vi "四台设备.vi"() -> ()   [LabVIEW 2012]
uses:
  <vilib>/Analysis/NI_AALPro.lvlib
panel:
  in  "选项卡控件 3":enum32{"振动", "振动 2", "转速", "温度湿度"}(tab)
  out "?":i16[](graph)
  out "?":i16[](graph)
  out "?":i16[](graph)
  out "?":i16[](graph)
  out "?":dbl[](graph)
  out "?":dbl[](graph)
  out "?":dbl[](graph)
  out "?":dbl[](graph)
  out "?":i16[](graph)
  out "?":dbl(graph)
  out "?":dbl(graph)
  out "?":dbl(graph)
  out "?":dbl(graph)
  out "?":u8(graph)
  out "?":u8(graph)
  out "?":dbl(graph)
  out "?":dbl(graph)
  in  "?":enum32{"振动", "振动 2", "转速", "温度湿度"}(tab)
  out "?":i16[](graph)
  out "?":i16[](graph)
  out "?":i16[](graph)
  out "?":i16[](graph)
  out "?":dbl[](graph)
  out "?":dbl[](graph)
  out "?":dbl[](graph)
  out "?":dbl[](graph)
  out "?":u16[](graph)
  out "?":dbl(graph)
  out "?":dbl(graph)
  out "?":u8(graph)
  out "?":dbl(graph)
  out "?":dbl(graph)
  out "?":u8(graph)
  out "?":dbl(graph)
  out "?":dbl(graph)
  in  "?":enum32{"振动", "振动 2", "转速", "温度湿度"}(tab)
  out "?":i16[](graph)
  out "?":i16[](graph)
  out "?":i16[](graph)
  out "?":i16[](graph)
  out "?":dbl[](graph)
  out "?":dbl[](graph)
  out "?":dbl[](graph)
  out "?":dbl[](graph)
  out "?":u16[](graph)
  out "?":dbl(graph)
  out "?":dbl(graph)
  out "?":dbl(graph)
  out "?":dbl(graph)
  out "?":dbl(graph)
  out "?":u8(graph)
  out "?":u8(graph)
  out "?":dbl(graph)
  out "KB/s 4":dbl
  out "收包 4":i32
  out "系统时间 4":string
  out "KB/s 3":dbl
  out "收包 3":i32
  out "系统时间 3":string
  out "KB/s 2":dbl
  out "收包 2":i32
  out "系统时间 2":string
  in  "?":enum32{"振动", "振动 2", "转速", "温度湿度"}(tab)
  out "?":i16[](graph)
  out "?":i16[](graph)
  out "?":i16[](graph)
  out "?":i16[](graph)
  out "?":dbl[](graph)
  out "?":dbl[](graph)
  out "?":dbl[](graph)
  out "?":dbl[](graph)
  out "?":u16[](graph)
  out "?":dbl(graph)
  out "?":dbl(graph)
  out "?":dbl(graph)
  out "?":dbl(graph)
  out "?":dbl(graph)
  out "?":dbl(graph)
  out "?":u8(graph)
  out "?":u8(graph)
  out "系统时间":string
  out "收包":i32
  out "KB/s":dbl
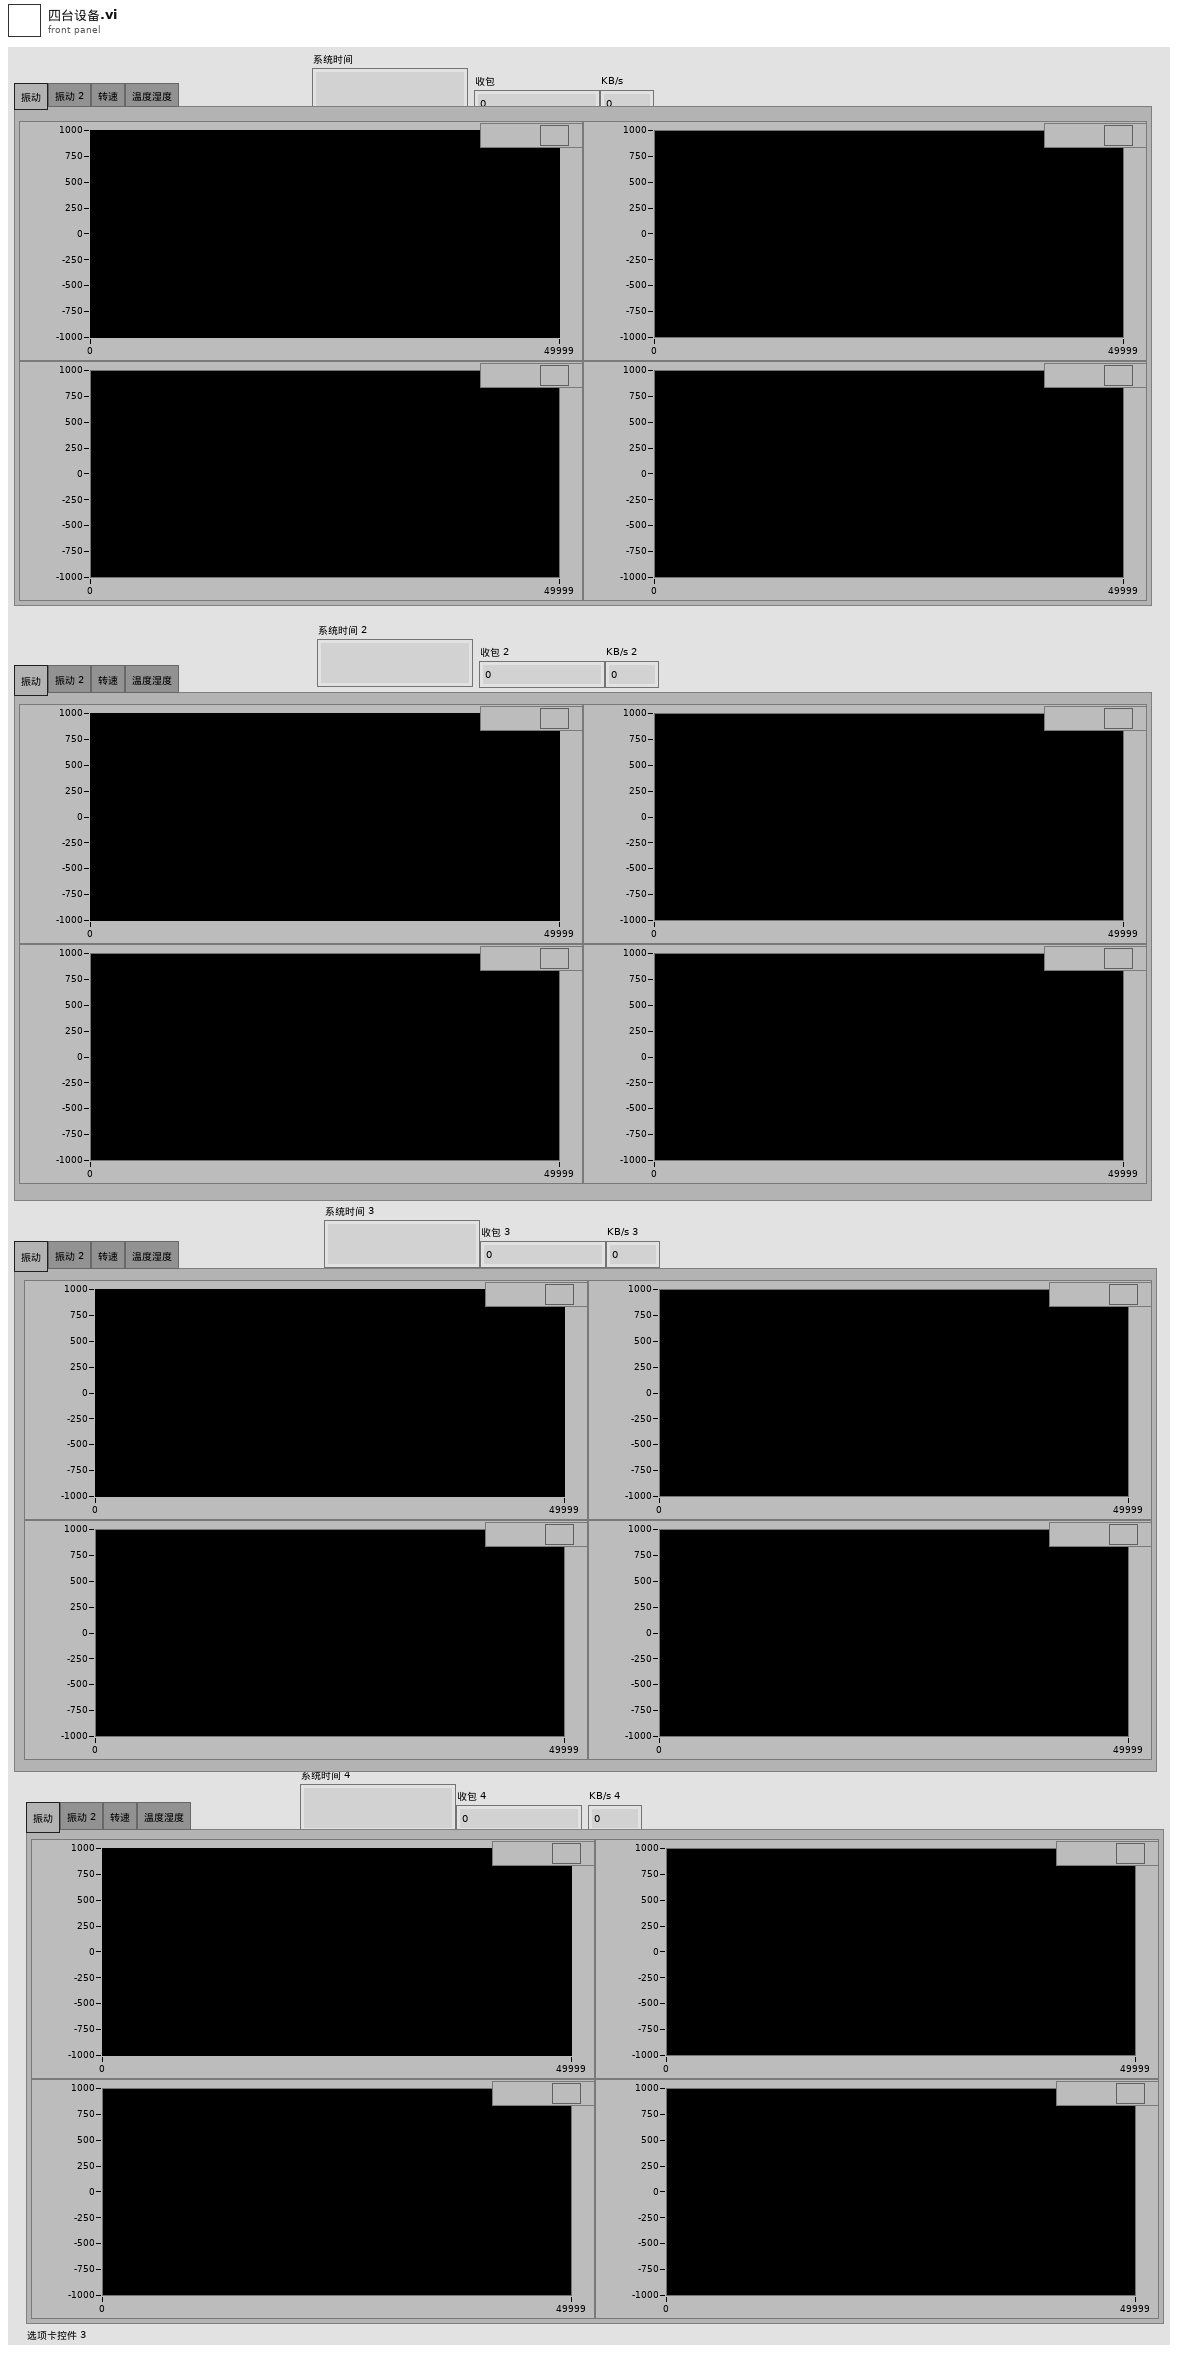
[diagram p1: front panel]
types:
  T1 = enum16{"open", "replace", "create", "open or create", "replace or create", "replace or create with confirmation"}
  T2 = enum16{"big-endian, network order", "native, host order", "little-endian"}
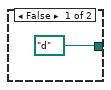
[diagram p2: hidden frame]
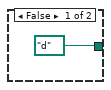
[diagram p3: hidden frame]
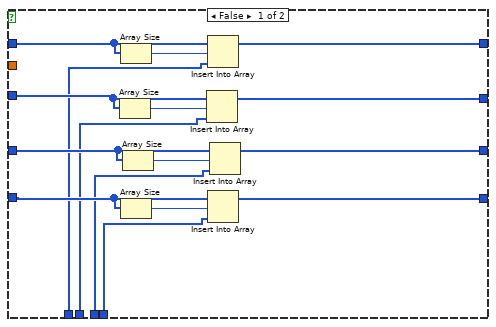
[diagram p4: hidden frame]
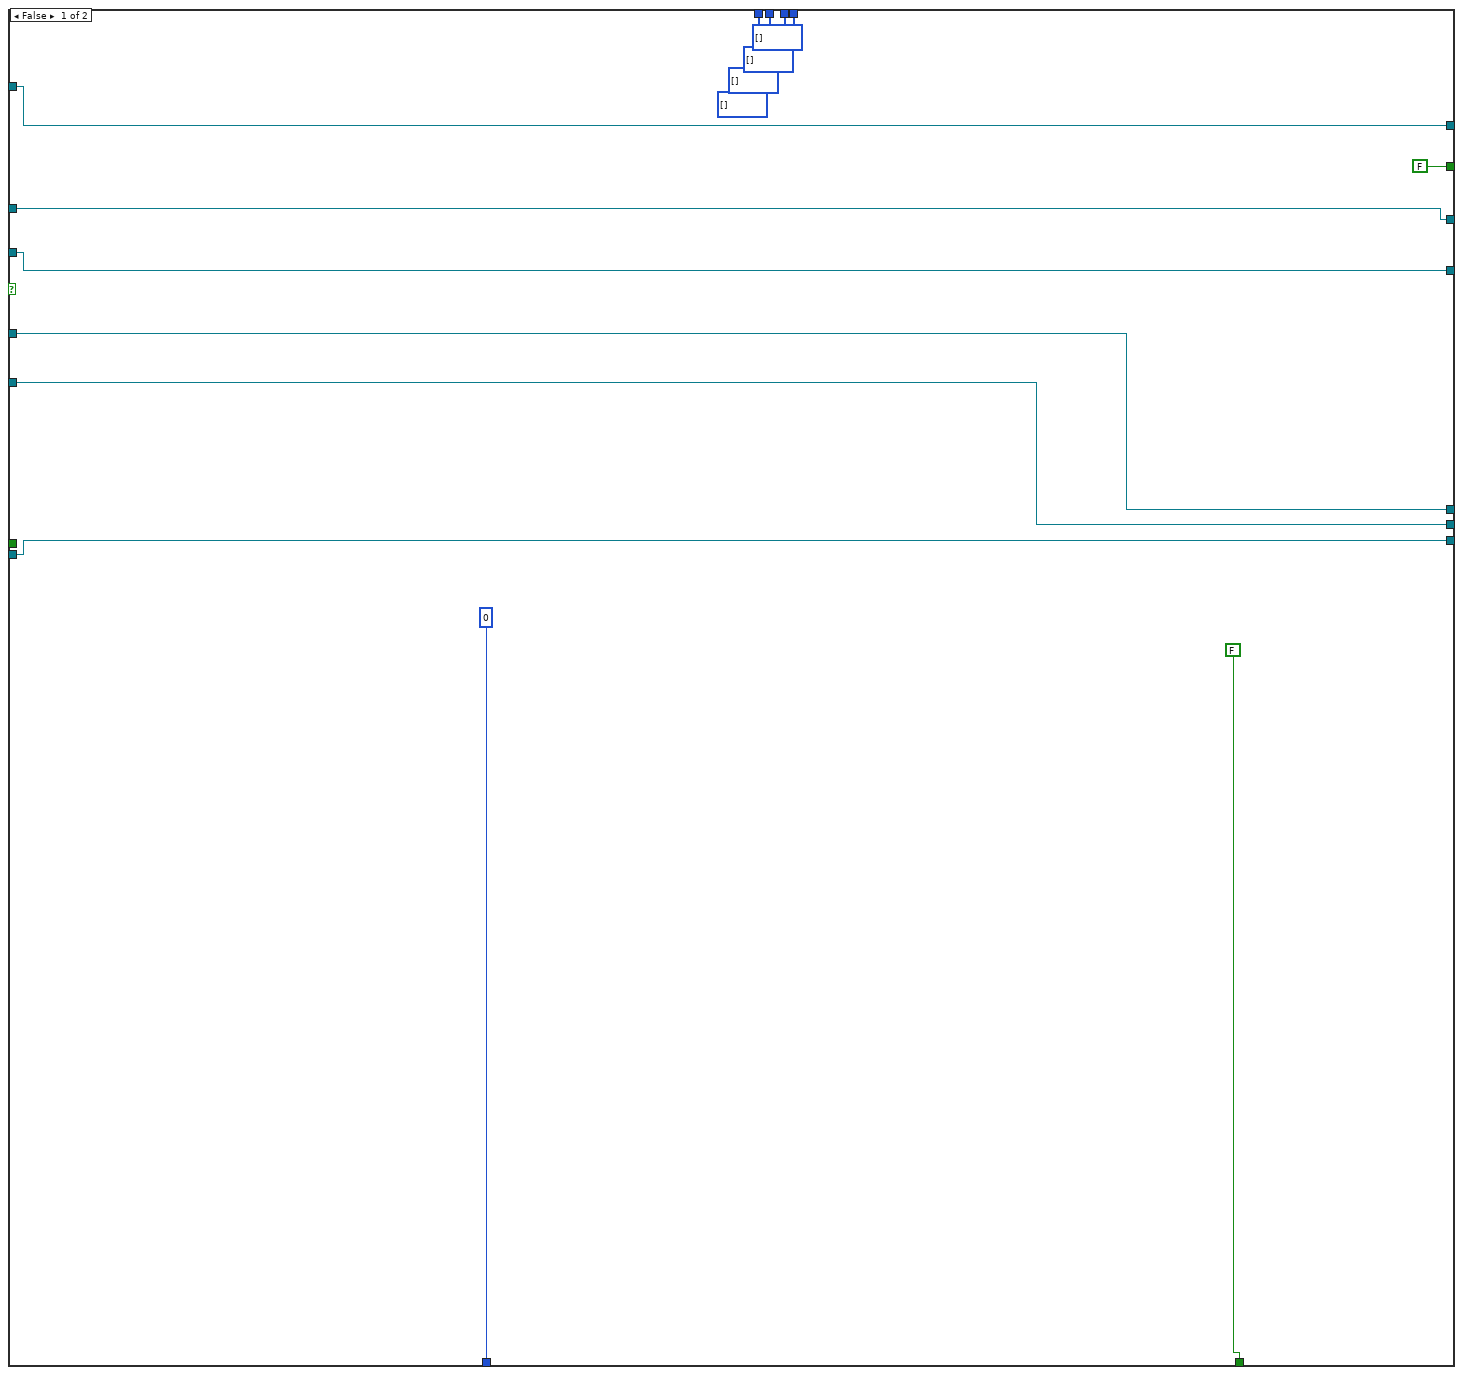
[diagram p5: hidden frame]
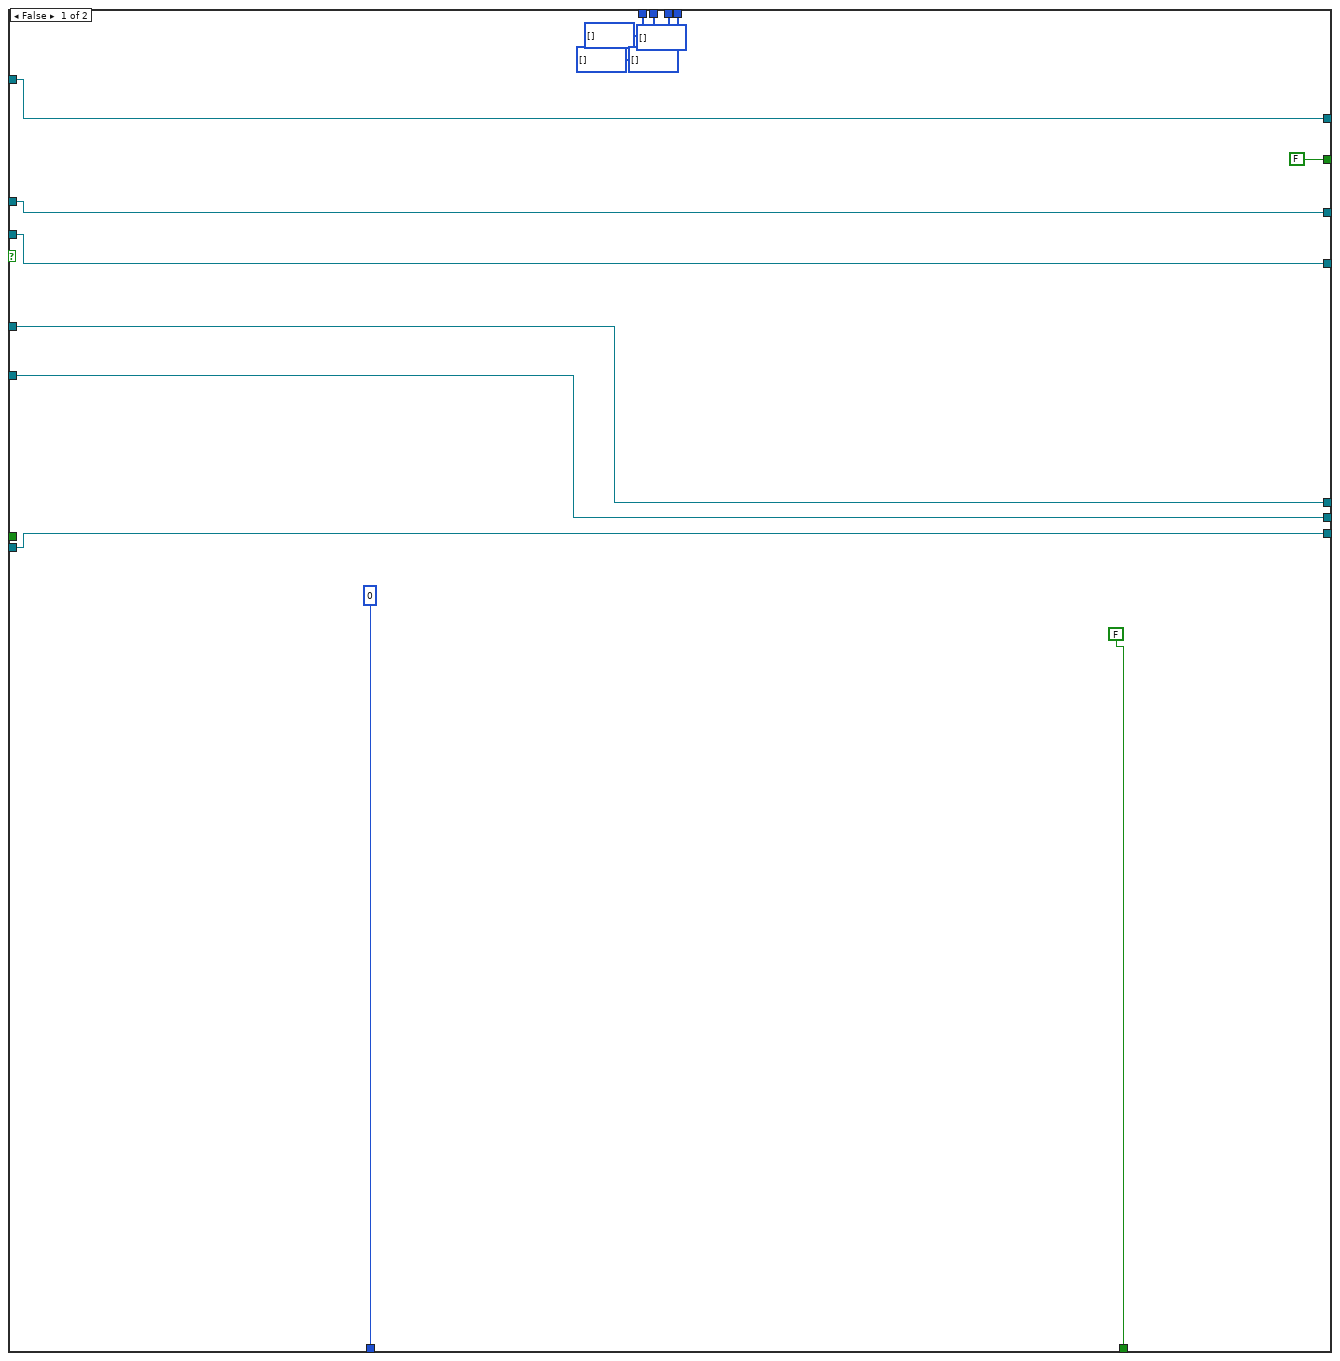
[diagram p6: hidden frame]
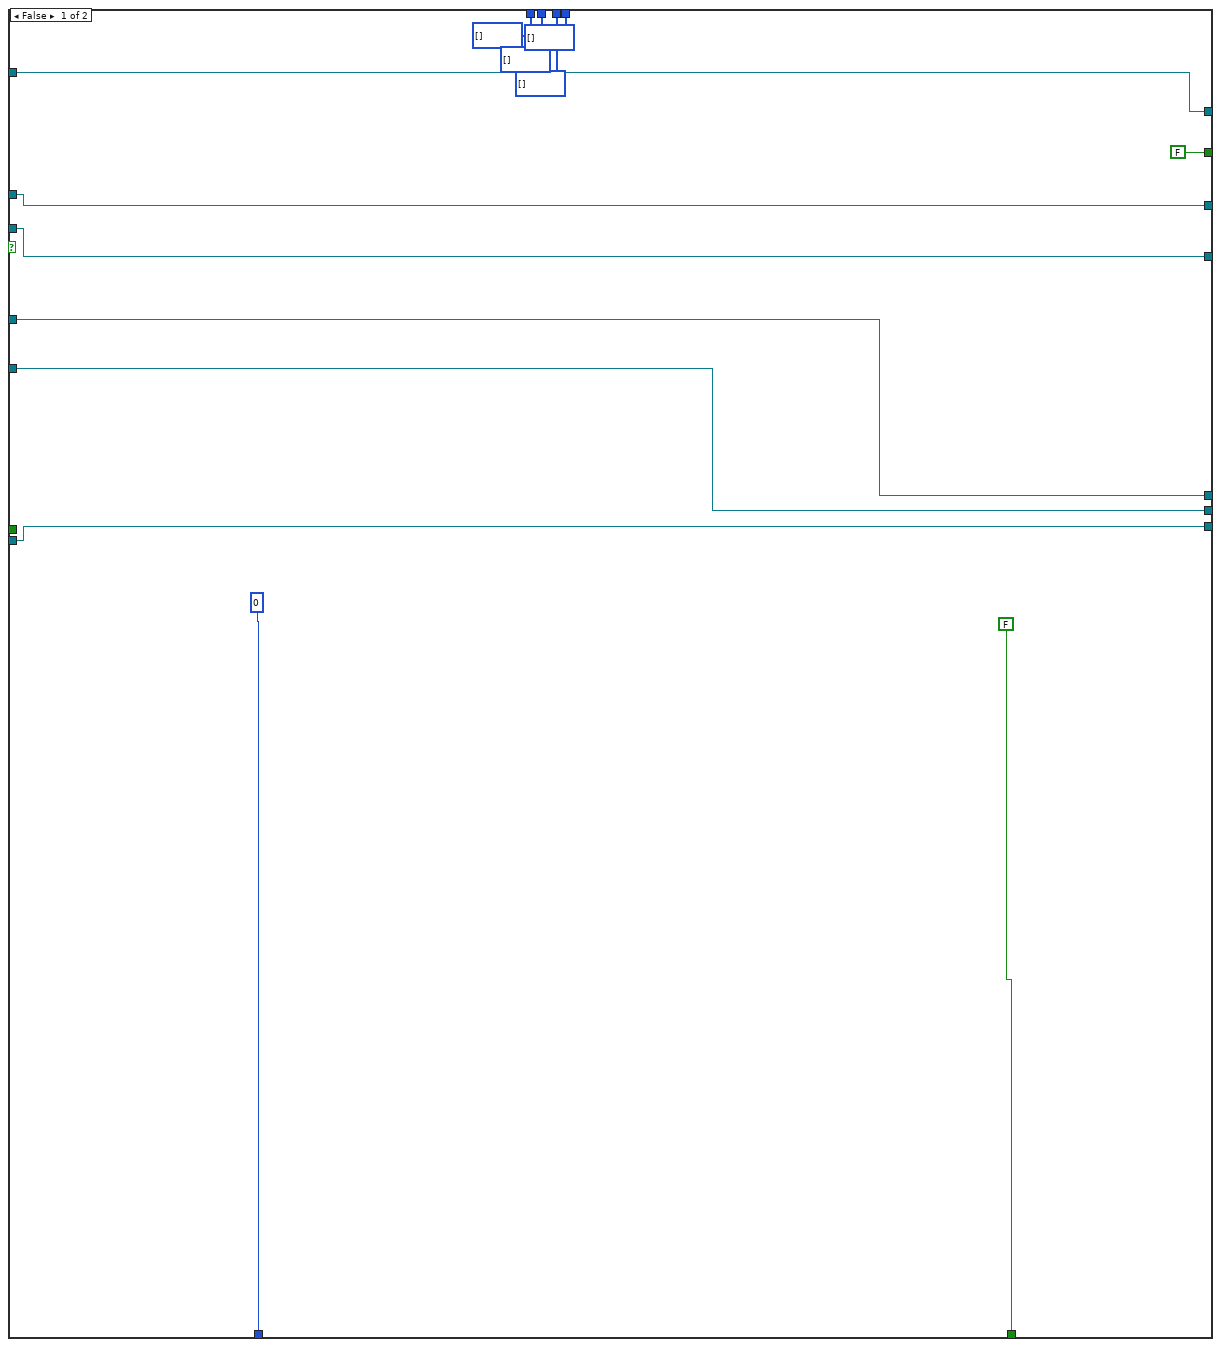
[diagram p7: hidden frame]
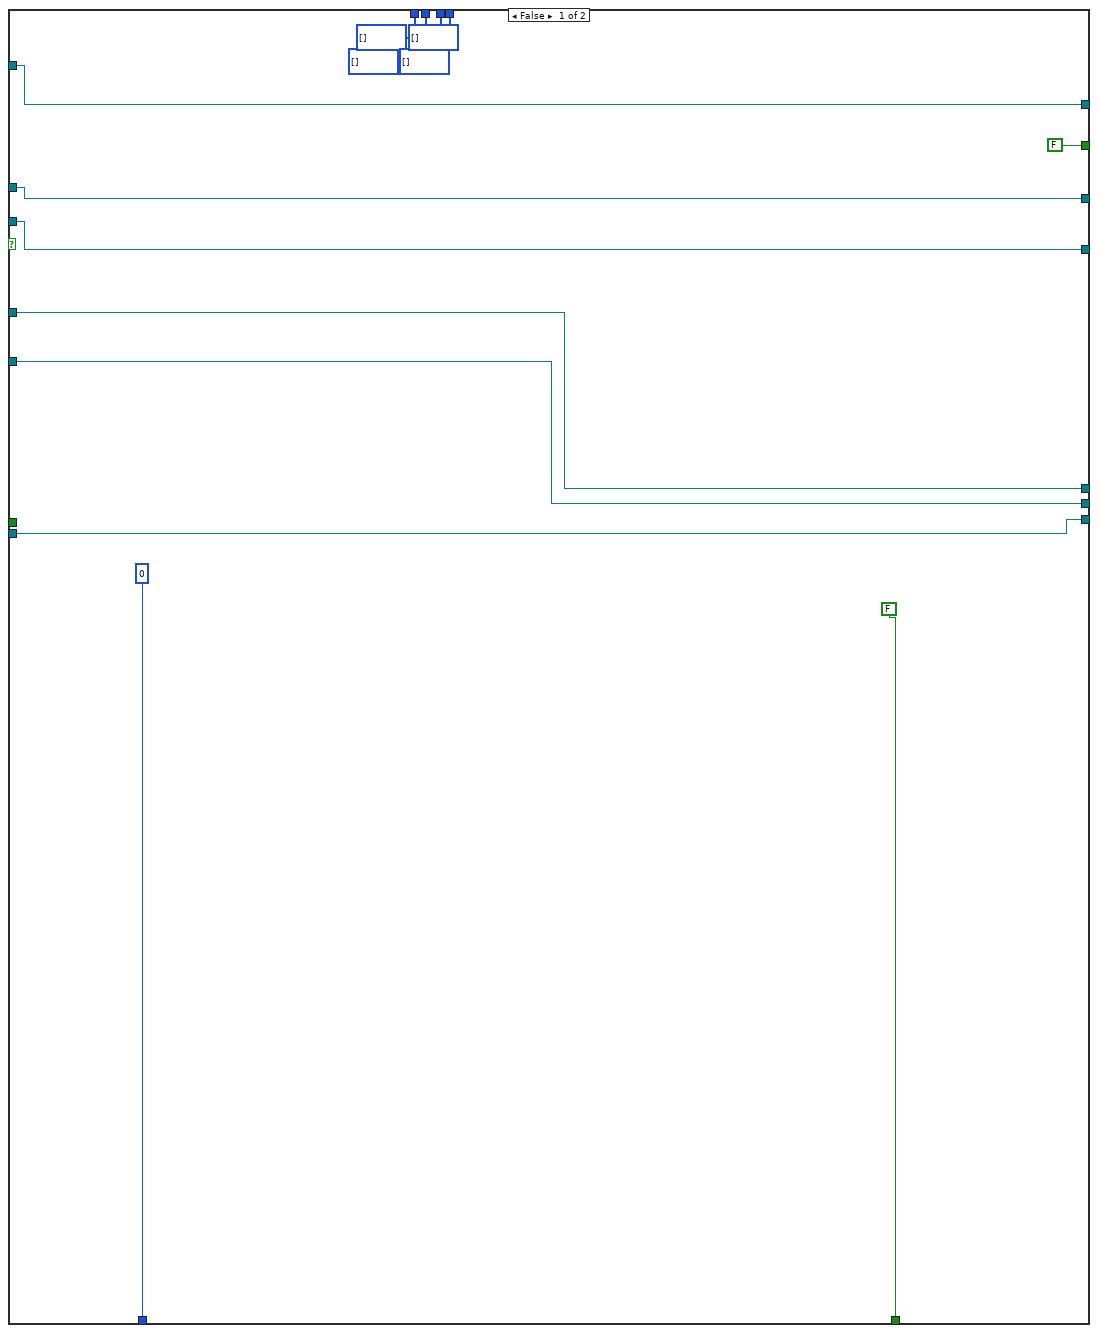
[diagram p8: hidden frame]
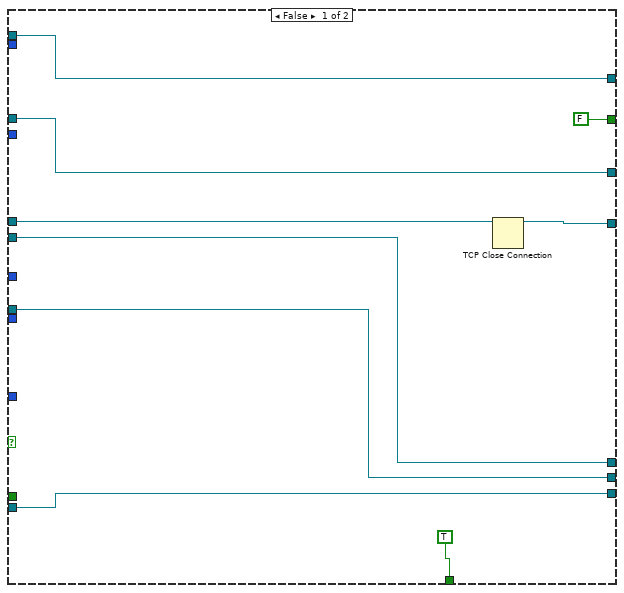
[diagram p9: hidden frame]
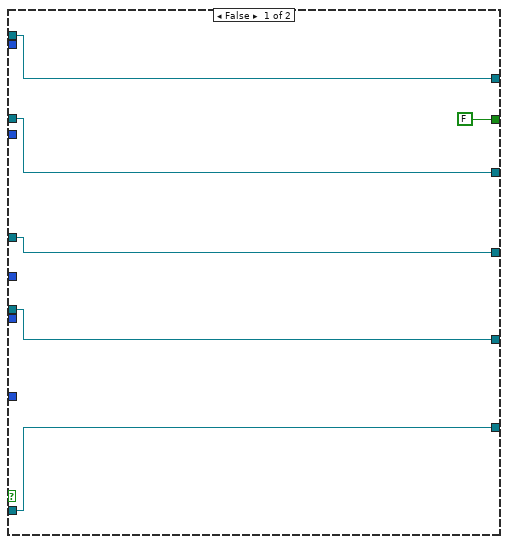
[diagram p10: hidden frame]
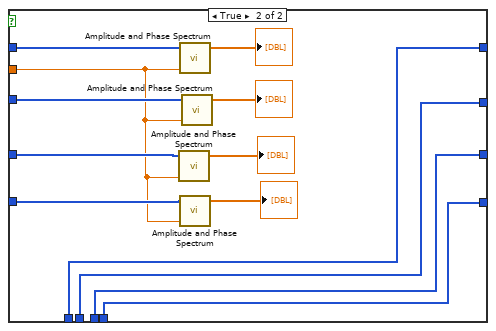
[diagram p12: hidden frame]
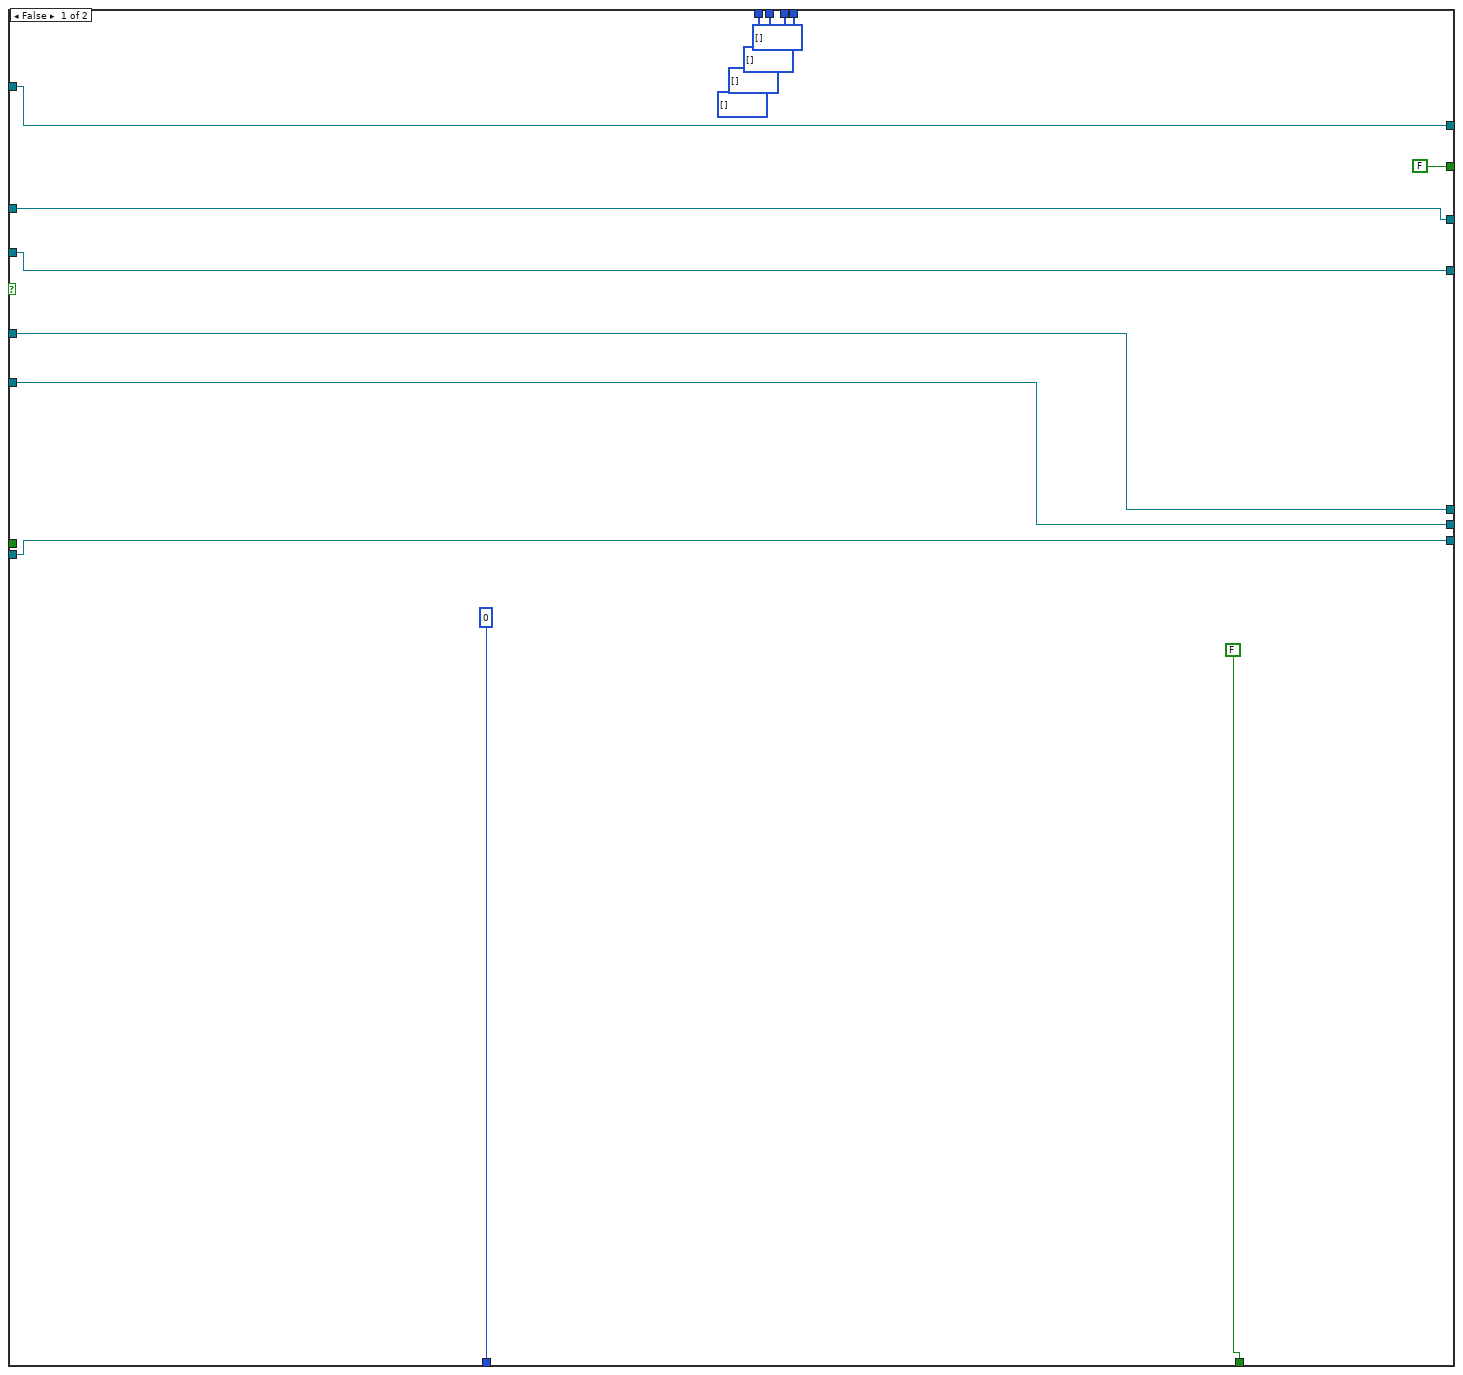
[diagram p13: hidden frame]
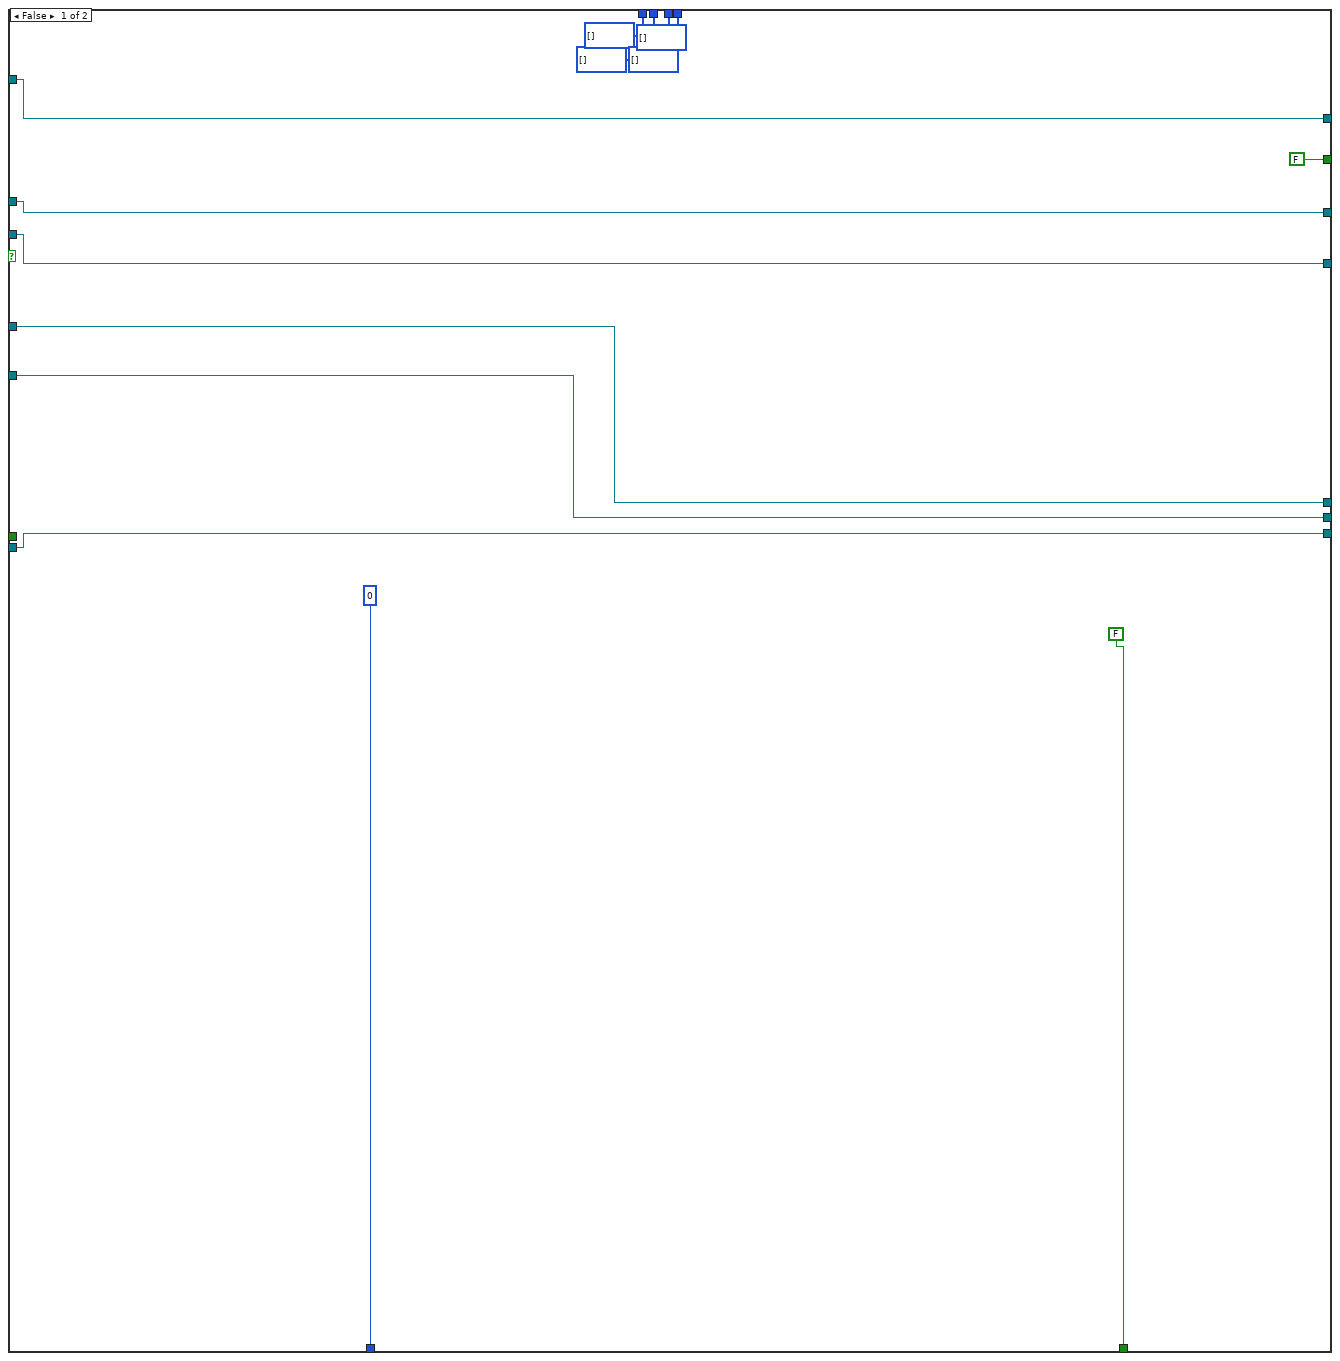
[diagram p14: hidden frame]
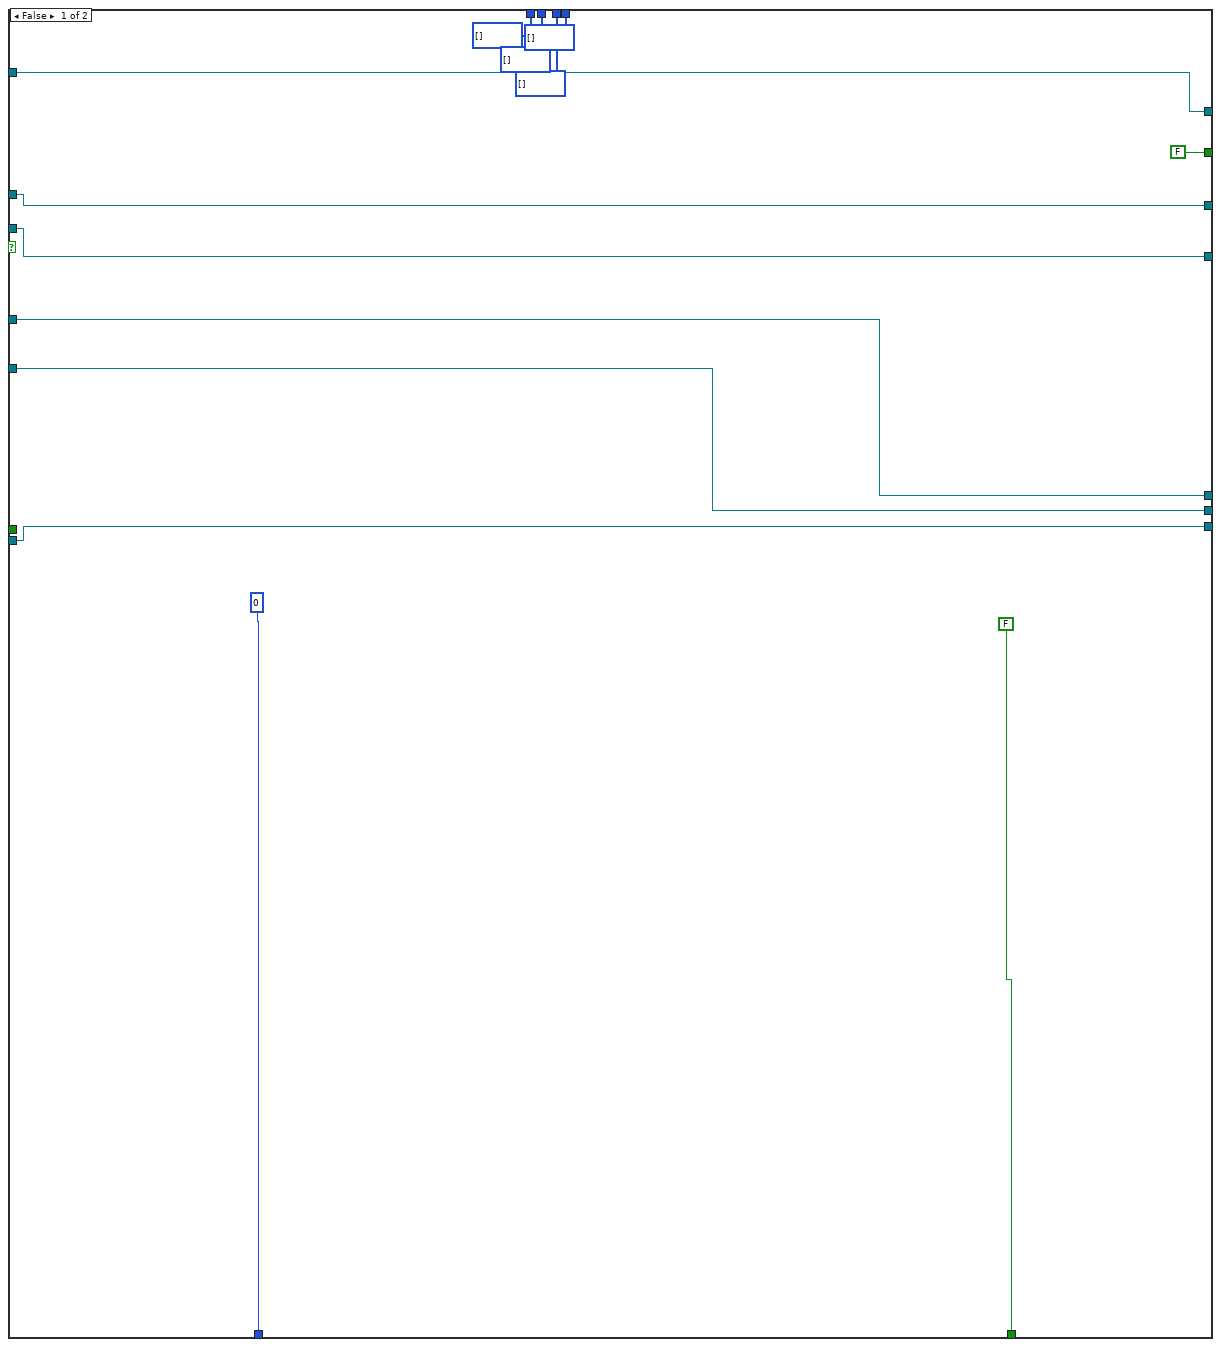
[diagram p15: hidden frame]
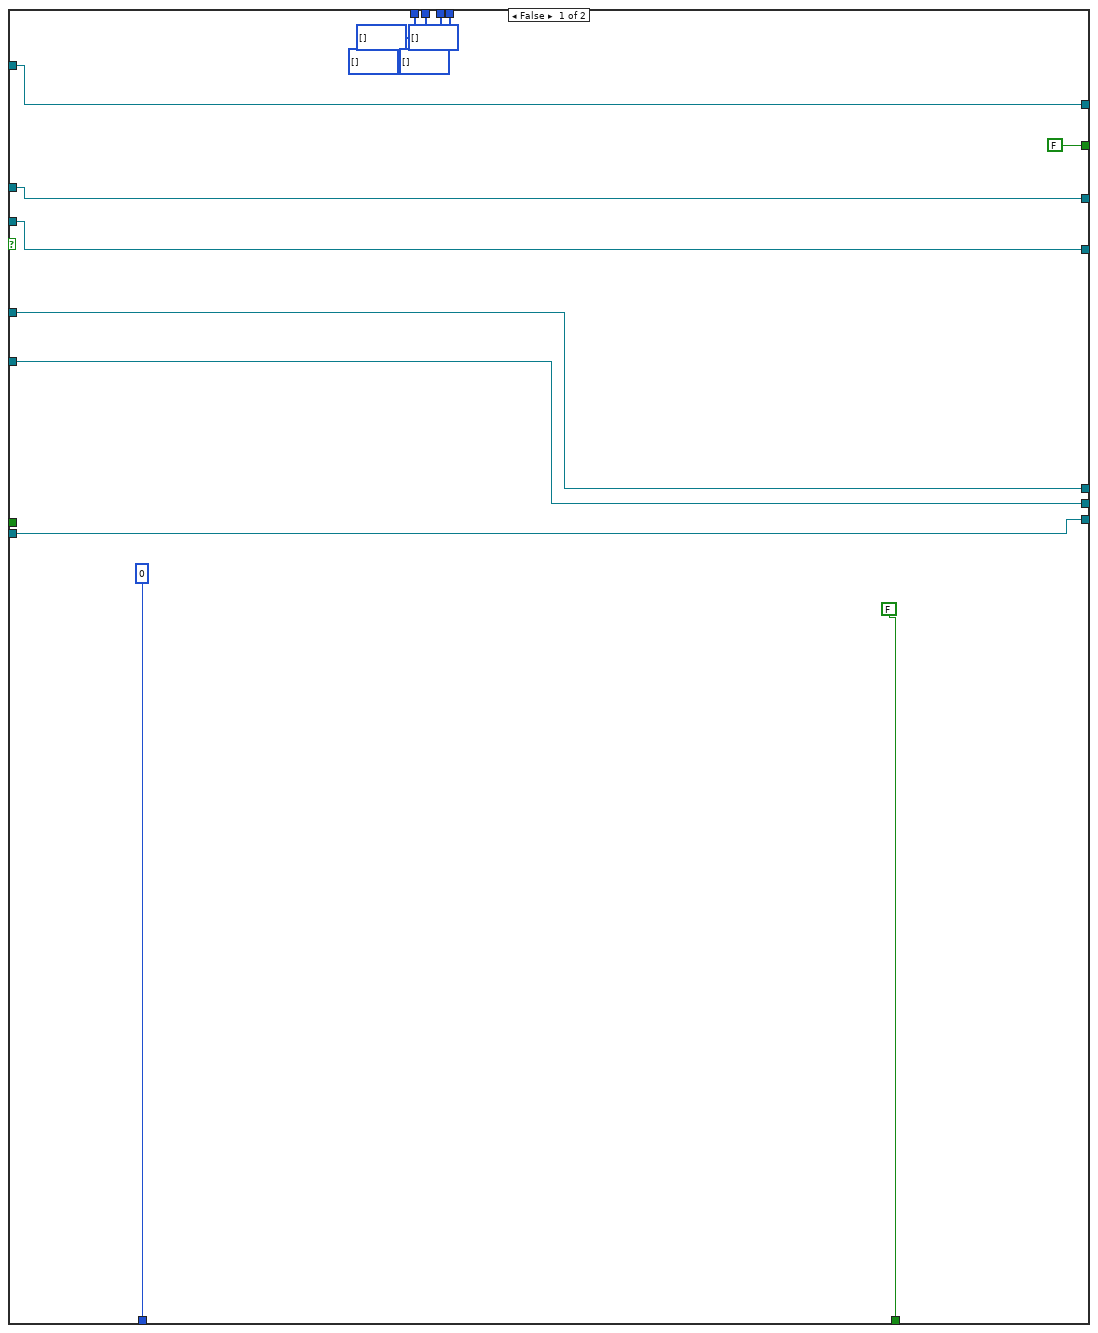
[diagram p16: hidden frame]
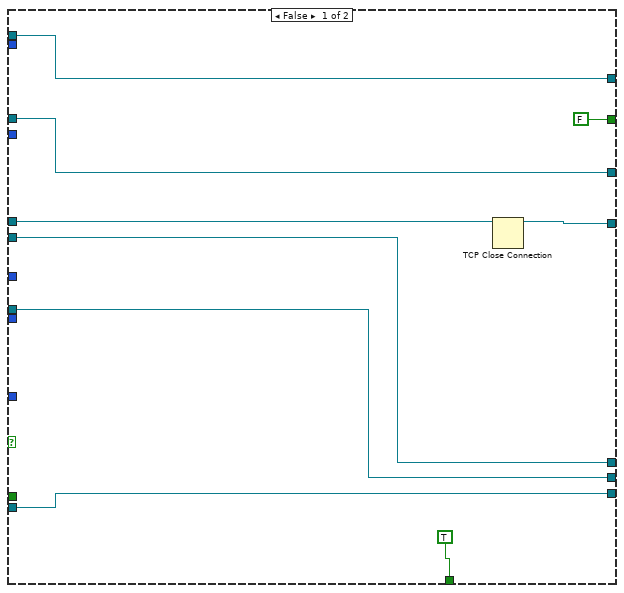
[diagram p17: hidden frame]
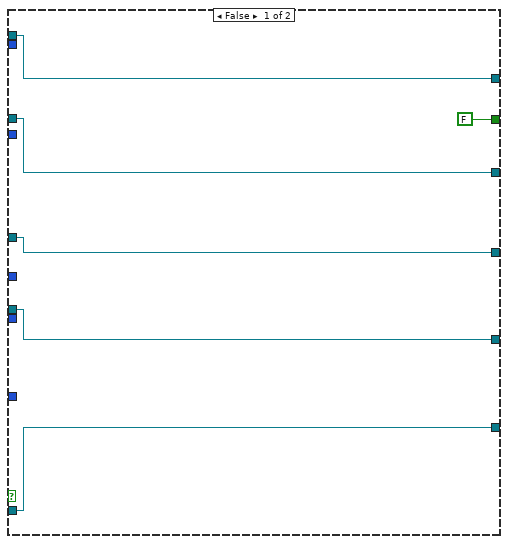
[diagram p18: hidden frame]
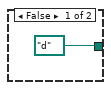
[diagram p20: hidden frame]
diagram:
  n1 = flat-sequence {
    tunnel: [w27] -> w18
    tunnel: [w21] -> w17
    tunnel: [w34] -> w19
    tunnel: [w33] -> w20
    frame #0 {
      n2 = call "分频系数"("Enable"=TRUE) -> ("#4分频系数"=w25:dbl, "#3分频系数"=w24:dbl, "#2分频系数"=w23:dbl, "#1分频系数"=w22:dbl, "总分频系数"=w26:dbl)  [unwired: 12 in, 2 out]
      n3 = To Unsigned Byte Integer(number=w26) -> (unsigned 8bit integer=w21:u8)
      n4 = To Unsigned Byte Integer(number=w25) -> (unsigned 8bit integer=w28:u8)
      n5 = To Unsigned Byte Integer(number=w22) -> (unsigned 8bit integer=w31:u8)
      n6 = To Unsigned Byte Integer(number=w23) -> (unsigned 8bit integer=w30:u8)
      n7 = To Unsigned Byte Integer(number=w24) -> (unsigned 8bit integer=w29:u8)
      n8 = Build Array(w21, w31, w30, w29, w28) -> (w27:u8[])
    }
    frame #1 {
      n9 = Two Button Dialog(message="是否储存数据" ("消息"), 1:"否" ("F按钮名称（“取消”）"), 2:"是" ("T按钮名称（“确定”）")) -> (T button?=w33:bool)
      n10 = case shown="真" w33 {
        tunnel: [path "d:/" ("路径（使用对话框）") w40] -> w34
        frame False {
        }
        frame True {
          n11 = Create Folder(prompt (Create Folder)="数据文件夹路径" ("对话框窗口（创建文件夹）")) -> (created path=w40:path)  [unwired: 2 in, 2 out]
        }
      }
    }
  }
  n12 = flat-sequence {
    tunnel: [w47] -> w1
    tunnel: [w41] -> w9
    tunnel: [w54] -> w3
    tunnel: [w53] -> w2
    frame #0 {
      n13 = call "分频系数4"("Enable"=TRUE) -> ("#4分频系数"=w45:dbl, "#3分频系数"=w44:dbl, "#2分频系数"=w43:dbl, "#1分频系数"=w42:dbl, "总分频系数"=w46:dbl)  [unwired: 12 in, 2 out]
      n14 = To Unsigned Byte Integer(number=w46) -> (unsigned 8bit integer=w41:u8)
      n15 = To Unsigned Byte Integer(number=w45) -> (unsigned 8bit integer=w48:u8)
      n16 = To Unsigned Byte Integer(number=w42) -> (unsigned 8bit integer=w51:u8)
      n17 = To Unsigned Byte Integer(number=w43) -> (unsigned 8bit integer=w50:u8)
      n18 = To Unsigned Byte Integer(number=w44) -> (unsigned 8bit integer=w49:u8)
      n19 = Build Array(w41, w51, w50, w49, w48) -> (w47:u8[])
    }
    frame #1 {
      n20 = Two Button Dialog(message="是否储存数据" ("消息"), 1:"否" ("F按钮名称（“取消”）"), 2:"是" ("T按钮名称（“确定”）")) -> (T button?=w53:bool)
      n21 = case shown="真" w53 {
        tunnel: [path "d:/" ("路径（使用对话框）") w60] -> w54
        frame False {
        }
        frame True {
          n22 = Create Folder(prompt (Create Folder)="数据文件夹路径" ("对话框窗口（创建文件夹）")) -> (created path=w60:path)  [unwired: 2 in, 2 out]
        }
      }
    }
  }
  n23 = flat-sequence {
    tunnel: [w67] -> w5
    tunnel: [w61] -> w10
    tunnel: [w74] -> w8
    tunnel: [w73] -> w7
    frame #0 {
      n24 = call "分频系数3"("Enable"=TRUE) -> ("#4分频系数"=w65:dbl, "#3分频系数"=w64:dbl, "#2分频系数"=w63:dbl, "#1分频系数"=w62:dbl, "总分频系数"=w66:dbl)  [unwired: 12 in, 2 out]
      n25 = To Unsigned Byte Integer(number=w66) -> (unsigned 8bit integer=w61:u8)
      n26 = To Unsigned Byte Integer(number=w65) -> (unsigned 8bit integer=w68:u8)
      n27 = To Unsigned Byte Integer(number=w62) -> (unsigned 8bit integer=w71:u8)
      n28 = To Unsigned Byte Integer(number=w63) -> (unsigned 8bit integer=w70:u8)
      n29 = To Unsigned Byte Integer(number=w64) -> (unsigned 8bit integer=w69:u8)
      n30 = Build Array(w61, w71, w70, w69, w68) -> (w67:u8[])
    }
    frame #1 {
      n31 = Two Button Dialog(message="是否储存数据" ("消息"), 1:"否" ("F按钮名称（“取消”）"), 2:"是" ("T按钮名称（“确定”）")) -> (T button?=w73:bool)
      n32 = case shown="真" w73 {
        tunnel: [path "d:/" ("路径（使用对话框）") w80] -> w74
        frame False {
        }
        frame True {
          n33 = Create Folder(prompt (Create Folder)="数据文件夹路径" ("对话框窗口（创建文件夹）")) -> (created path=w80:path)  [unwired: 2 in, 2 out]
        }
      }
    }
  }
  n34 = flat-sequence {
    tunnel: [w87] -> w12
    tunnel: [w81] -> w15
    tunnel: [w94] -> w14
    tunnel: [w93] -> w13
    frame #0 {
      n35 = call "分频系数2"("Enable"=TRUE) -> ("#4分频系数"=w85:dbl, "#3分频系数"=w84:dbl, "#2分频系数"=w83:dbl, "#1分频系数"=w82:dbl, "总分频系数"=w86:dbl)  [unwired: 12 in, 2 out]
      n36 = To Unsigned Byte Integer(number=w86) -> (unsigned 8bit integer=w81:u8)
      n37 = To Unsigned Byte Integer(number=w85) -> (unsigned 8bit integer=w88:u8)
      n38 = To Unsigned Byte Integer(number=w82) -> (unsigned 8bit integer=w91:u8)
      n39 = To Unsigned Byte Integer(number=w83) -> (unsigned 8bit integer=w90:u8)
      n40 = To Unsigned Byte Integer(number=w84) -> (unsigned 8bit integer=w89:u8)
      n41 = Build Array(w81, w91, w90, w89, w88) -> (w87:u8[])
    }
    frame #1 {
      n42 = Two Button Dialog(message="是否储存数据" ("消息"), 1:"否" ("F按钮名称（“取消”）"), 2:"是" ("T按钮名称（“确定”）")) -> (T button?=w93:bool)
      n43 = case shown="真" w93 {
        tunnel: [path "d:/" ("路径（使用对话框）") w100] -> w94
        frame False {
        }
        frame True {
          n44 = Create Folder(prompt (Create Folder)="数据文件夹路径" ("对话框窗口（创建文件夹）")) -> (created path=w100:path)  [unwired: 2 in, 2 out]
        }
      }
    }
  }
  n45 = Increment(x=w17) -> (x+1=w16:u8)
  n46 = Increment(x=w9) -> (x+1=w4:u8)
  n47 = Increment(x=w10) -> (x+1=w6:u8)
  n48 = Increment(x=w15) -> (x+1=w11:u8)
  n49 = while {
    tunnel: w20 -> [w153]
    tunnel: w19 -> [w152]
    tunnel: w18 -> [w138]
    tunnel: w16 -> [w151]
    stop <- FALSE stop-if-true
    n50 = Split 1D Array(array=w138, index=1 ("索引")) -> (first subarray=w136:u8[], second subarray=w132:u8[])
    n51 = Split 1D Array(array=w132, index=1 ("索引")) -> (first subarray=w112:u8[], second subarray=w131:u8[])
    n52 = Split 1D Array(array=w131, index=1 ("索引")) -> (first subarray=w111:u8[], second subarray=w130:u8[])
    n53 = Split 1D Array(array=w130, index=1 ("索引")) -> (first subarray=w110:u8[], second subarray=w109:u8[])
    n54 = flat-sequence {
      tunnel: [w157] -> w102
      tunnel: w102 -> [w161]
      tunnel: [w159] -> w101
      frame #0 {
        n55 = Wait (ms)(milliseconds to wait=u32 1000 ("毫秒倍数")) -> ()  [unwired: 1 out]
      }
      frame #1 {
        n56 = TCP Open Connection(address="192.168.1.15" ("名称"), remote port or service name=u16 3855 ("端口")) -> (connection ID=w157:refnum<k5>)  [unwired: 3 in, 1 out]
      }
      frame #2 {
        n57 = TCP Write(connection ID=w161, data in="INTxxxxx" ("数据输入")) -> (connection ID out=w160:refnum<k5>)  [unwired: 2 in, 2 out]
        n58 = while {
          tunnel: w160 -> [w170]
          tunnel: [w164] -> w159
          stop <- w165 stop-if-true
          n59 = TCP Read(connection ID=w170, bytes to read=8 ("读取的字节")) -> (connection ID out=w164:refnum<k5>, data out=w168:string)  [unwired: 3 in, 1 out]
          n60 = String Subset(string=w168, length (rest)=3 ("偏移量(0)")) -> (substring=w167:string)  [unwired: 1 in]
          n61 = Equal?(x=w167, y="ACK") -> (x = y?=w165:bool)
        }
      }
    }
    n62 = Byte Array To String(unsigned byte array=w136) -> (string=w141:string)
    n63 = Byte Array To String(unsigned byte array=u8[] [3] ("无符号字节数组")) -> (string=w118:string)
    n64 = Byte Array To String(unsigned byte array=u8[] [1] ("无符号字节数组")) -> (string=w126:string)
    n65 = Byte Array To String(unsigned byte array=w110) -> (string=w120:string)
    n66 = Byte Array To String(unsigned byte array=w112) -> (string=w129:string)
    n67 = Concatenate Strings("PRExxxx" ("数据输入"), w141) -> (w139:string)
    n68 = Concatenate Strings("DIVxxx" ("数据输入"), w126, w129) -> (w128:string)
    n69 = Concatenate Strings("DIVxxx" ("数据输入"), w118, w120) -> (w103:string)
    n70 = TCP Write(connection ID=w101, data in=w139) -> (connection ID out=w150:refnum<k5>)  [unwired: 2 in, 2 out]
    n71 = while {
      tunnel: w150 -> [w210]
      tunnel: [w204] -> w145
      stop <- w205 stop-if-true
      n72 = TCP Read(connection ID=w210, bytes to read=8 ("读取的字节")) -> (connection ID out=w204:refnum<k5>, data out=w208:string)  [unwired: 3 in, 1 out]
      n73 = String Subset(string=w208, length (rest)=3 ("偏移量(0)")) -> (substring=w207:string)  [unwired: 1 in]
      n74 = Equal?(x=w207, y="ACK") -> (x = y?=w205:bool)
    }
    n75 = TCP Write(connection ID=w145, data in=w128) -> (connection ID out=w149:refnum<k5>)  [unwired: 2 in, 2 out]
    n76 = while {
      tunnel: w149 -> [w202]
      tunnel: [w196] -> w144
      stop <- w197 stop-if-true
      n77 = TCP Read(connection ID=w202, bytes to read=8 ("读取的字节")) -> (connection ID out=w196:refnum<k5>, data out=w200:string)  [unwired: 3 in, 1 out]
      n78 = String Subset(string=w200, length (rest)=3 ("偏移量(0)")) -> (substring=w199:string)  [unwired: 1 in]
      n79 = Equal?(x=w199, y="ACK") -> (x = y?=w197:bool)
    }
    n80 = Byte Array To String(unsigned byte array=u8[] [4] ("无符号字节数组")) -> (string=w114:string)
    n81 = Byte Array To String(unsigned byte array=w109) -> (string=w116:string)
    n82 = Byte Array To String(unsigned byte array=u8[] [2] ("无符号字节数组")) -> (string=w122:string)
    n83 = Byte Array To String(unsigned byte array=w111) -> (string=w124:string)
    n84 = Concatenate Strings("DIVxxx" ("数据输入"), w114, w116) -> (w107:string)
    n85 = Concatenate Strings("DIVxxx" ("数据输入"), w122, w124) -> (w108:string)
    n86 = TCP Write(connection ID=w144, data in=w108) -> (connection ID out=w148:refnum<k5>)  [unwired: 2 in, 2 out]
    n87 = while {
      tunnel: w148 -> [w194]
      tunnel: [w188] -> w143
      stop <- w189 stop-if-true
      n88 = TCP Read(connection ID=w194, bytes to read=8 ("读取的字节")) -> (connection ID out=w188:refnum<k5>, data out=w192:string)  [unwired: 3 in, 1 out]
      n89 = String Subset(string=w192, length (rest)=3 ("偏移量(0)")) -> (substring=w191:string)  [unwired: 1 in]
      n90 = Equal?(x=w191, y="ACK") -> (x = y?=w189:bool)
    }
    n91 = TCP Write(connection ID=w143, data in=w103) -> (connection ID out=w147:refnum<k5>)  [unwired: 2 in, 2 out]
    n92 = while {
      tunnel: w147 -> [w186]
      tunnel: [w180] -> w142
      stop <- w181 stop-if-true
      n93 = TCP Read(connection ID=w186, bytes to read=8 ("读取的字节")) -> (connection ID out=w180:refnum<k5>, data out=w184:string)  [unwired: 3 in, 1 out]
      n94 = String Subset(string=w184, length (rest)=3 ("偏移量(0)")) -> (substring=w183:string)  [unwired: 1 in]
      n95 = Equal?(x=w183, y="ACK") -> (x = y?=w181:bool)
    }
    n96 = TCP Write(connection ID=w142, data in=w107) -> (connection ID out=w146:refnum<k5>)  [unwired: 2 in, 2 out]
    n97 = while {
      tunnel: w146 -> [w178]
      tunnel: [w172] -> w106
      stop <- w173 stop-if-true
      n98 = TCP Read(connection ID=w178, bytes to read=8 ("读取的字节")) -> (connection ID out=w172:refnum<k5>, data out=w176:string)  [unwired: 3 in, 1 out]
      n99 = String Subset(string=w176, length (rest)=3 ("偏移量(0)")) -> (substring=w175:string)  [unwired: 1 in]
      n100 = Equal?(x=w175, y="ACK") -> (x = y?=w173:bool)
    }
    n101 = TCP Write(connection ID=w106, data in="STAxxxxx" ("数据输入")) -> (connection ID out=w104:refnum<k5>)  [unwired: 2 in, 2 out]
    n102 = while {
      tunnel: w104 -> [w259]
      tunnel: w153 -> [w258]
      tunnel: w152 -> [w231]
      tunnel: w151 -> [w211]
      stop <- w221 stop-if-true
      n103 = Get Date/Time String(want seconds? (F)=TRUE ("需要秒？(F)")) -> (date string=w229:string, time string=w226:string)  [unwired: 2 in]
      n104 = Concatenate Strings(w229, "-" ("字符串"), w226, ".bin" ("字符串")) -> (w225:string)
      n105 = Path To String(path=w231) -> (string=w242:string)
      n106 = Search and Replace String(replace all?=TRUE ("替换全部？(F)"), input string=w225, search string=":" ("搜索字符串"), replace string="-" ("替换字符串(\"\")")) -> (result string=w217:string)  [unwired: 4 in, 3 out]
      n107 = Search and Replace String(replace all?=TRUE ("替换全部？(F)"), input string=w217, search string="/" ("搜索字符串"), replace string="-" ("替换字符串(\"\")")) -> (result string=w216:string)  [unwired: 4 in, 3 out]
      n108 = Concatenate Strings(w242, "\\振动2-" ("字符串"), w216) -> (w249:string)
      n109 = Concatenate Strings(w242, "\\振动1-" ("字符串"), w216) -> (w248:string)
      n110 = Concatenate Strings(w242, "\\振动4-" ("字符串"), w216) -> (w251:string)
      n111 = Concatenate Strings(w242, "\\振动3-" ("字符串"), w216) -> (w250:string)
      n112 = Concatenate Strings(w242, "\\转速-" ("字符串"), w216) -> (w252:string)
      n113 = String To Path(string=w249) -> (path=w246:path)
      n114 = String To Path(string=w250) -> (path=w245:path)
      n115 = String To Path(string=w248) -> (path=w247:path)
      n116 = String To Path(string=w251) -> (path=w244:path)
      n117 = String To Path(string=w252) -> (path=w243:path)
      n118 = Open/Create/Replace File(file path (use dialog)=w244, operation (0:open)=T1."open or create" ("操作(0:open)")) -> (refnum out=w233:refnum<file>)  [unwired: 4 in, 2 out]
      n119 = Open/Create/Replace File(file path (use dialog)=w246, operation (0:open)=T1."open or create" ("操作(0:open)")) -> (refnum out=w235:refnum<file>)  [unwired: 4 in, 2 out]
      n120 = Open/Create/Replace File(file path (use dialog)=w245, operation (0:open)=T1."open or create" ("操作(0:open)")) -> (refnum out=w234:refnum<file>)  [unwired: 4 in, 2 out]
      n121 = Open/Create/Replace File(file path (use dialog)=w243, operation (0:open)=T1."open or create" ("操作(0:open)")) -> (refnum out=w232:refnum<file>)  [unwired: 4 in, 2 out]
      n122 = Open/Create/Replace File(file path (use dialog)=w247, operation (0:open)=T1."open or create" ("操作(0:open)")) -> (refnum out=w236:refnum<file>)  [unwired: 4 in, 2 out]
      n123 = while {
        shift-right: [w317] -> _
        shift-left: _ -> [w316]
        shift-right: [w299] -> _
        shift-left: w259 -> [w303]
        shift-right: [w311] -> _
        shift-left: _ -> [w314]
        shift-right: [w308] -> _
        shift-left: _ -> [w309]
        shift-right: [w306] -> _
        shift-left: _ -> [w304]
        shift-right: [w295] -> _
        shift-left: w236 -> [w290]
        shift-right: [w294] -> _
        shift-left: w235 -> [w289]
        shift-right: [w293] -> _
        shift-left: w234 -> [w288]
        shift-right: [w292] -> _
        shift-left: w233 -> [w287]
        shift-right: [w291] -> _
        shift-left: w232 -> [w286]
        tunnel: w258 -> [w285]
        tunnel: [w283] -> w221
        shift-right: [w267] -> _
        shift-left: i16[] [] -> [w271]
        shift-right: [w268] -> _
        shift-left: i16[] [] -> [w272]
        shift-right: [w269] -> _
        shift-left: i16[] [] -> [w273]
        shift-right: [w270] -> _
        shift-left: i16[] [] -> [w266]
        tunnel: w211 -> [w262]
        i -> [w281]
        stop <- w282 stop-if-true
        n124 = TCP Read(connection ID=w303, bytes to read=1 ("读取的字节")) -> (connection ID out=w296:refnum<k5>, data out=w301:string)  [unwired: 3 in, 1 out]
        n125 = Equal?(x=w301, y="D") -> (x = y?=w297:bool)
        n126 = case shown="真" w297 {
          tunnel: w296 -> [w359 w380]
          tunnel: [w359 w379] -> w299
          tunnel: [0 w378] -> w298
          tunnel: [FALSE w376] -> w283
          tunnel: [w356 w375] -> w295
          tunnel: [w355 w368] -> w294
          tunnel: [w354 w367] -> w293
          tunnel: [w353 w366] -> w292
          tunnel: [w352 w374] -> w291
          tunnel: w290 -> [w356 w373]
          tunnel: w289 -> [w355 w372]
          tunnel: w288 -> [w354 w371]
          tunnel: w287 -> [w353 w370]
          tunnel: w286 -> [w352 w369]
          tunnel: w285 -> [_ w365]
          tunnel: [FALSE w364] -> w284
          tunnel: [i16[] [] w363] -> w277
          tunnel: [i16[] [] w362] -> w276
          tunnel: [i16[] [] w361] -> w275
          tunnel: [i16[] [] w360] -> w274
          frame False {
          }
          frame True {
            n127 = TCP Read(connection ID=w380, bytes to read=1 ("读取的字节")) -> (connection ID out=w377:refnum<k5>, data out=w383:string)  [unwired: 3 in, 1 out]
            n128 = Equal?(x=w383, y="A") -> (x = y?=w381:bool)
            n129 = case shown="真" w381 {
              tunnel: w377 -> [w397 w418]
              tunnel: [w397 w417] -> w379
              tunnel: [0 w416] -> w378
              tunnel: [FALSE w414] -> w376
              tunnel: [w394 w413] -> w375
              tunnel: [w390 w409] -> w374
              tunnel: w373 -> [w394 w408]
              tunnel: w372 -> [w393 w407]
              tunnel: w371 -> [w392 w406]
              tunnel: w370 -> [w391 w405]
              tunnel: w369 -> [w390 w404]
              tunnel: [w393 w412] -> w368
              tunnel: [w392 w411] -> w367
              tunnel: [w391 w410] -> w366
              tunnel: w365 -> [_ w403]
              tunnel: [FALSE w402] -> w364
              tunnel: [i16[] [] w401] -> w363
              tunnel: [i16[] [] w400] -> w362
              tunnel: [i16[] [] w399] -> w361
              tunnel: [i16[] [] w398] -> w360
              frame False {
              }
              frame True {
                n130 = TCP Read(connection ID=w418, bytes to read=1 ("读取的字节")) -> (connection ID out=w415:refnum<k5>, data out=w421:string)  [unwired: 3 in, 1 out]
                n131 = Equal?(x=w421, y="T") -> (x = y?=w419:bool)
                n132 = case shown="真" w419 {
                  tunnel: w415 -> [w435 w457]
                  tunnel: [w435 w454] -> w417
                  tunnel: [0 w456] -> w416
                  tunnel: [FALSE w453] -> w414
                  tunnel: [w428 w445] -> w413
                  tunnel: [w429 w444] -> w412
                  tunnel: [w430 w443] -> w411
                  tunnel: [w431 w452] -> w410
                  tunnel: [w432 w451] -> w409
                  tunnel: w408 -> [w428 w450]
                  tunnel: w407 -> [w429 w449]
                  tunnel: w406 -> [w430 w448]
                  tunnel: w405 -> [w431 w447]
                  tunnel: w404 -> [w432 w446]
                  tunnel: w403 -> [_ w442]
                  tunnel: [FALSE w441] -> w402
                  tunnel: [i16[] [] w440] -> w401
                  tunnel: [i16[] [] w439] -> w400
                  tunnel: [i16[] [] w438] -> w399
                  tunnel: [i16[] [] w437] -> w398
                  frame False {
                  }
                  frame True {
                    n133 = TCP Read(connection ID=w457, bytes to read=2 ("读取的字节")) -> (connection ID out=w455:refnum<k5>)  [unwired: 3 in, 2 out]
                    n134 = case shown="真" TRUE {
                      tunnel: w455 -> [w471 w607]
                      tunnel: [0 w598] -> w456
                      tunnel: [w471 w591] -> w454
                      tunnel: [FALSE w592] -> w453
                      tunnel: [w465 w574] -> w452
                      tunnel: [w464 w573] -> w451
                      tunnel: w450 -> [w468 w580]
                      tunnel: w449 -> [w467 w578]
                      tunnel: w448 -> [w466 w576]
                      tunnel: w447 -> [w465 w500]
                      tunnel: w446 -> [w464 w572]
                      tunnel: [w468 w579] -> w445
                      tunnel: [w467 w577] -> w444
                      tunnel: [w466 w575] -> w443
                      tunnel: w442 -> [_ w570]
                      tunnel: [FALSE w568] -> w441
                      tunnel: [i16[] [] w499] -> w440
                      tunnel: [i16[] [] w498] -> w439
                      tunnel: [i16[] [] w497] -> w438
                      tunnel: [i16[] [] w496] -> w437
                      frame False {
                      }
                      frame True {
                        n135 = TCP Read(connection ID=w607, bytes to read=4021 ("最大值(548)")) -> (connection ID out=w581:refnum<k5>, data out=w590:string)  [unwired: 3 in, 1 out]
                        n136 = String To Byte Array(string=w590) -> (unsigned byte array=w589:u8[])
                        n137 = String Length(string=w590) -> (length=w598:i32)
                        n138 = Split 1D Array(array=w589, index=1000 ("索引")) -> (first subarray=w494:u8[], second subarray=w491:u8[])
                        n139 = Split 1D Array(array=w491, index=1000 ("索引")) -> (first subarray=w490:u8[], second subarray=w487:u8[])
                        n140 = Split 1D Array(array=w487, index=1000 ("索引")) -> (first subarray=w486:u8[], second subarray=w485:u8[])
                        n141 = Split 1D Array(array=w485, index=1000 ("索引")) -> (first subarray=w482:u8[], second subarray=w495:u8[])
                        n142 = Split 1D Array(array=w495, index=2 ("索引")) -> (first subarray=w475:u8[], second subarray=w567:u8[])
                        n143 = Split 1D Array(array=w567, index=2 ("索引")) -> (first subarray=w550:u8[], second subarray=w566:u8[])
                        n144 = Split 1D Array(array=w566, index=2 ("索引")) -> (first subarray=w514:u8[], second subarray=w565:u8[])
                        n145 = Split 1D Array(array=w565, index=2 ("索引")) -> (first subarray=w513:u8[], second subarray=w552:u8[])
                        n146 = Split 1D Array(array=w552, index=2 ("索引")) -> (first subarray=w512:u8[], second subarray=w561:u8[])
                        n147 = Split 1D Array(array=w561, index=2 ("索引")) -> (first subarray=w511:u8[], second subarray=w560:u8[])
                        n148 = Split 1D Array(array=w560, index=2 ("索引")) -> (first subarray=w510:u8[], second subarray=w551:u8[])
                        n149 = Split 1D Array(array=w551, index=2 ("索引")) -> (first subarray=w509:u8[], second subarray=w473:u8[])
                        n150 = Split 1D Array(array=w473, index=5 ("索引")) -> (first subarray=w472:u8[])  [unwired: 1 out]
                        n151 = Decimate 1D Array(w494) -> (w493:u8[], w492:u8[])
                        n152 = Decimate 1D Array(w490) -> (w489:u8[], w488:u8[])
                        n153 = Decimate 1D Array(w486) -> (w484:u8[], w483:u8[])
                        n154 = Decimate 1D Array(w482) -> (w481:u8[], w480:u8[])
                        n155 = Decimate 1D Array(w475) -> (w477:u8[], w476:u8[])
                        n156 = Get Date/Time String(date format (0)=enum16{"short", "long", "abbreviated"}."short" ("日期格式(0)"), want seconds? (F)=TRUE ("需要秒？(F)")) -> (date string=w586:string, time string=w569:string)  [unwired: 1 in]
                        n157 = Join Numbers(hi=w477, lo=w476) -> ((hi.lo)=w479:u16[])
                        n158 = Join Numbers(hi=w493, lo=w492) -> ((hi.lo)=w605:u16[])
                        n159 = Join Numbers(hi=w489, lo=w488) -> ((hi.lo)=w600:u16[])
                        n160 = Join Numbers(hi=w484, lo=w483) -> ((hi.lo)=w601:u16[])
                        n161 = Join Numbers(hi=w481, lo=w480) -> ((hi.lo)=w602:u16[])
                        n162 = Index Array(array=w550, index=0 ("索引")) -> (element=w545:u8)
                        n163 = Index Array(array=w550, index=1 ("索引")) -> (element=w547:u8)
                        n164 = String To Byte Array(string="_PSAI") -> (unsigned byte array=w595:u8[])
                        n165 = Index Array(array=w514, index=0 ("索引")) -> (element=w539:u8)
                        n166 = Index Array(array=w514, index=1 ("索引")) -> (element=w541:u8)
                        n167 = Index Array(array=w512, index=0 ("索引")) -> (element=w527:u8)
                        n168 = Index Array(array=w513, index=0 ("索引")) -> (element=w533:u8)
                        n169 = Index Array(array=w512, index=1 ("索引")) -> (element=w529:u8)
                        n170 = Index Array(array=w513, index=1 ("索引")) -> (element=w535:u8)
                        n171 = Index Array(array=w511, index=0 ("索引")) -> (element=w521:u8)
                        n172 = To Word Integer(number=w605) -> (16bit integer=w499:i16[])
                        "?" <- w499
                        n173 = Index Array(array=w511, index=1 ("索引")) -> (element=w523:u8)
                        n174 = To Unsigned Word Integer(number=w479) -> (unsigned 16bit integer=w478:u16[])
                        "?" <- w478
                        n175 = To Word Integer(number=w600) -> (16bit integer=w498:i16[])
                        "?" <- w498
                        n176 = Index Array(array=w510, index=0 ("索引")) -> (element=w515:u8)
                        n177 = call <vilib>:"Space Constant.vi"() -> ("String"=w582:string)
                        n178 = Index Array(array=w510, index=1 ("索引")) -> (element=w517:u8)
                        n179 = To Word Integer(number=w601) -> (16bit integer=w497:i16[])
                        "?" <- w497
                        n180 = To Word Integer(number=w602) -> (16bit integer=w496:i16[])
                        "?" <- w496
                        n181 = Equal?(x=w472, y=w595) -> (x = y?=w594:bool[])
                        n182 = Index Array(array=w509, index=0 ("索引")) -> (element=→"?":u8)
                        n183 = Divide(x=w547, y=10.0) -> (x/y=w546:dbl)
                        n184 = Divide(x=w541, y=10.0) -> (x/y=w540:dbl)
                        n185 = Divide(x=w529, y=10.0) -> (x/y=w528:dbl)
                        n186 = Divide(x=w535, y=10.0) -> (x/y=w534:dbl)
                        n187 = Concatenate Strings("\r", "@@" ("字符串"), w586, w582, w569, "@@" ("字符串")) -> (w585:string)
                        "系统时间" <- w585
                        n188 = Divide(x=w523, y=10.0) -> (x/y=w522:dbl)
                        n189 = Index Array(array=w509, index=1 ("索引")) -> (element=→"?":u8)
                        n190 = Divide(x=w517, y=10.0) -> (x/y=w516:dbl)
                        n191 = And Array Elements(Boolean array=w594) -> (logical AND=w593:bool)
                        n192 = Add(x=w545, y=w546) -> (x+y=→"?":dbl)
                        n193 = Add(x=w539, y=w540) -> (x+y=→"?":dbl)
                        n194 = Add(x=w527, y=w528) -> (x+y=→"?":dbl)
                        n195 = Add(x=w533, y=w534) -> (x+y=→"?":dbl)
                        n196 = Add(x=w521, y=w522) -> (x+y=→"?":dbl)
                        n197 = Add(x=w515, y=w516) -> (x+y=→"?":dbl)
                        n198 = local write "系统时间"(w585) -> ()
                        n199 = case shown="真" w593 {
                          tunnel: [w617 w636] -> w591
                          tunnel: [TRUE FALSE] -> w592
                          tunnel: w581 -> [w615 w636]
                          tunnel: w499 -> [_ w635]
                          tunnel: w498 -> [_ w634]
                          tunnel: w497 -> [_ w633]
                          tunnel: w496 -> [_ w632]
                          tunnel: w478 -> [_ w631]
                          tunnel: w580 -> [w613 w629]
                          tunnel: [w613 w628] -> w579
                          tunnel: w578 -> [w614 w627]
                          tunnel: [w614 w626] -> w577
                          tunnel: w576 -> [w612 w625]
                          tunnel: [w612 w624] -> w575
                          tunnel: w500 -> [w611 w623]
                          tunnel: [w611 w622] -> w574
                          tunnel: [w610 w621] -> w573
                          tunnel: w572 -> [w610 w620]
                          tunnel: w570 -> [_ w619]
                          tunnel: [FALSE w618] -> w568
                          frame False {
                            n200 = TCP Close Connection(connection ID=w615) -> (connection ID out=w617:refnum<k5>)  [unwired: 2 in, 1 out]
                          }
                          frame True {
                            n201 = case shown="真" w619 {
                              tunnel: w635 -> [_ w689]
                              tunnel: w634 -> [_ w669]
                              tunnel: w633 -> [_ w668]
                              tunnel: w632 -> [_ w667]
                              tunnel: w631 -> [_ w666]
                              tunnel: w629 -> [w642 w655]
                              tunnel: [w642 w646] -> w628
                              tunnel: w627 -> [w641 w654]
                              tunnel: [w641 w653] -> w626
                              tunnel: w625 -> [w640 w652]
                              tunnel: [w640 w647] -> w624
                              tunnel: w623 -> [w639 w651]
                              tunnel: [w639 w650] -> w622
                              tunnel: [w638 w649] -> w621
                              tunnel: w620 -> [w638 w648]
                              tunnel: [FALSE w643] -> w618
                              frame False {
                              }
                              frame True {
                                n202 = local read "系统时间"() -> (w663:string)
                                n203 = local read "系统时间"() -> (w665:string)
                                n204 = local read "系统时间"() -> (w657:string)
                                n205 = local read "系统时间"() -> (w659:string)
                                n206 = local read "系统时间"() -> (w661:string)
                                n207 = String To Byte Array(string=w663) -> (unsigned byte array=w662:u8[])
                                n208 = String To Byte Array(string=w659) -> (unsigned byte array=w658:u8[])
                                n209 = String To Byte Array(string=w657) -> (unsigned byte array=w656:u8[])
                                n210 = String To Byte Array(string=w665) -> (unsigned byte array=w664:u8[])
                                n211 = String To Byte Array(string=w661) -> (unsigned byte array=w660:u8[])
                                n212 = Insert Into Array(array=w689, index=0 ("索引"), new element=w656) -> (w687:i16[])
                                n213 = Insert Into Array(array=w669, index=0 ("索引"), new element=w658) -> (w683:i16[])
                                n214 = Insert Into Array(array=w668, index=0 ("索引"), new element=w660) -> (w679:i16[])
                                n215 = Insert Into Array(array=w667, index=0 ("索引"), new element=w662) -> (w675:i16[])
                                n216 = Insert Into Array(array=w666, index=0 ("索引"), new element=w664) -> (w671:u16[])
                                n217 = Write to Binary File(file (use dialog)=w655, data=w687, 5:FALSE ("预置数组或字符串大小？(T)"), 9:T2."little-endian" ("字节顺序(0:big-endian, network order)")) -> (refnum out=w646:refnum<file>)  [unwired: 2 in, 2 out]
                                n218 = Write to Binary File(file (use dialog)=w654, data=w683, 5:FALSE ("预置数组或字符串大小？(T)"), 9:T2."little-endian" ("字节顺序(0:big-endian, network order)")) -> (refnum out=w653:refnum<file>)  [unwired: 2 in, 2 out]
                                n219 = Write to Binary File(file (use dialog)=w652, data=w679, 5:FALSE ("预置数组或字符串大小？(T)"), 9:T2."little-endian" ("字节顺序(0:big-endian, network order)")) -> (refnum out=w647:refnum<file>)  [unwired: 2 in, 2 out]
                                n220 = Write to Binary File(file (use dialog)=w651, data=w675, 5:FALSE ("预置数组或字符串大小？(T)"), 9:T2."little-endian" ("字节顺序(0:big-endian, network order)")) -> (refnum out=w650:refnum<file>)  [unwired: 2 in, 2 out]
                                n221 = Write to Binary File(file (use dialog)=w648, data=w671, 5:FALSE ("预置数组或字符串大小？(T)"), 9:T2."little-endian" ("字节顺序(0:big-endian, network order)")) -> (refnum out=w649:refnum<file>)  [unwired: 2 in, 2 out]
                                n222 = Get File Size(file=w646) -> (size (in bytes)=w645:i64)  [unwired: 1 in, 2 out]
                                n223 = Greater Or Equal?(x=w645, y=i64 60000000) -> (x >= y?=w643:bool)
                              }
                            }
                          }
                        }
                      }
                    }
                  }
                }
              }
            }
          }
        }
        n224 = Divide(x=u8 187, y=w262) -> (x/y=w260:dbl)
        n225 = Round Toward -Infinity(1:w260) -> (0:w264:dbl)
        n226 = Multiply(x=w264, y=500.0) -> (x*y=w263:dbl)
        n227 = Quotient & Remainder(x=w281, y=w264) -> (x-y*floor(x/y)=w280:dbl)  [unwired: 1 out]
        n228 = Equal?(x=w280, y=0) -> (x = y?=w278:bool)
        n229 = case shown="真" w278 {
          tunnel: w277 -> [w321 w346]
          tunnel: w276 -> [w320 w345]
          tunnel: w275 -> [w319 w344]
          tunnel: w274 -> [w318 w343]
          tunnel: [w329 w346] -> w267
          tunnel: [w328 w345] -> w268
          tunnel: [w327 w344] -> w269
          tunnel: [w326 w343] -> w270
          tunnel: w266 -> [w325 w339]
          tunnel: w273 -> [w324 w342]
          tunnel: w272 -> [w323 w340]
          tunnel: w271 -> [w322 w341]
          tunnel: w263 -> [_ w334]
          frame False {
            n230 = Array Size(array=w324) -> (size(s)=w331:i32)
            n231 = Array Size(array=w325) -> (size(s)=w330:i32)
            n232 = Array Size(array=w322) -> (size(s)=w333:i32)
            n233 = Array Size(array=w323) -> (size(s)=w332:i32)
            n234 = Insert Into Array(array=w324, index=w331, new element=w319) -> (w327:i16[])
            n235 = Insert Into Array(array=w325, index=w330, new element=w318) -> (w326:i16[])
            n236 = Insert Into Array(array=w322, index=w333, new element=w321) -> (w329:i16[])
            n237 = Insert Into Array(array=w323, index=w332, new element=w320) -> (w328:i16[])
          }
          frame True {
            n238 = call <vilib>:"Amplitude and Phase Spectrum.vi"("dt"=w334, "Signal (V)"=w340) -> ("Amp Spectrum Mag (Vrms)"=→"?":dbl[])  [unwired: 1 in, 2 out]
            n239 = call <vilib>:"Amplitude and Phase Spectrum.vi"("dt"=w334, "Signal (V)"=w339) -> ("Amp Spectrum Mag (Vrms)"=→"?":dbl[])  [unwired: 1 in, 2 out]
            n240 = call <vilib>:"Amplitude and Phase Spectrum.vi"("dt"=w334, "Signal (V)"=w341) -> ("Amp Spectrum Mag (Vrms)"=→"?":dbl[])  [unwired: 1 in, 2 out]
            n241 = call <vilib>:"Amplitude and Phase Spectrum.vi"("dt"=w334, "Signal (V)"=w342) -> ("Amp Spectrum Mag (Vrms)"=→"?":dbl[])  [unwired: 1 in, 2 out]
          }
        }
        n242 = Add(x=w316, y=w298) -> (x+y=w317:i32)
        "收包" <- w317
        n243 = Tick Count (ms)() -> (millisecond timer value=w308:u32)
        n244 = Subtract(x=w308, y=w309) -> (x-y=w307:u32)
        n245 = Subtract(x=w317, y=w316) -> (x-y=w315:i32)
        n246 = Add(x=w315, y=w314) -> (x+y=w310:i32)
        n247 = Add(x=w304, y=w307) -> (x+y=w305:u32)
        n248 = Greater Or Equal?(x=w310, y=1000000) -> (x >= y?=w312:bool)
        n249 = Or(x=w284, y=w283) -> (x .or. y?=w282:bool)
        n250 = case shown="真" w312 {
          tunnel: [w692 0] -> w311
          tunnel: w310 -> [w692 w695]
          tunnel: [w691 u32 0] -> w306
          tunnel: w305 -> [w691 w696]
          frame False {
          }
          frame True {
            n251 = Divide(x=w695, y=w696) -> (x/y=→"KB/s":dbl)
          }
        }
      }
    }
  }
  n252 = while {
    tunnel: w13 -> [w750]
    tunnel: w14 -> [w749]
    tunnel: w12 -> [w735]
    tunnel: w11 -> [w748]
    stop <- FALSE stop-if-true
    n253 = Split 1D Array(array=w735, index=1 ("索引")) -> (first subarray=w733:u8[], second subarray=w729:u8[])
    n254 = Split 1D Array(array=w729, index=1 ("索引")) -> (first subarray=w709:u8[], second subarray=w728:u8[])
    n255 = Split 1D Array(array=w728, index=1 ("索引")) -> (first subarray=w708:u8[], second subarray=w727:u8[])
    n256 = Split 1D Array(array=w727, index=1 ("索引")) -> (first subarray=w707:u8[], second subarray=w706:u8[])
    n257 = flat-sequence {
      tunnel: [w753] -> w699
      tunnel: w699 -> [w758]
      tunnel: [w756] -> w698
      frame #0 {
        n258 = Wait (ms)(milliseconds to wait=u32 1000 ("毫秒倍数")) -> ()  [unwired: 1 out]
      }
      frame #1 {
        n259 = TCP Open Connection(address="192.168.1.16" ("名称"), remote port or service name=u16 3856 ("端口")) -> (connection ID=w753:refnum<k5>)  [unwired: 3 in, 1 out]
      }
      frame #2 {
        n260 = TCP Write(connection ID=w758, data in="INTxxxxx" ("数据输入")) -> (connection ID out=w757:refnum<k5>)  [unwired: 2 in, 2 out]
        n261 = while {
          tunnel: w757 -> [w767]
          tunnel: [w761] -> w756
          stop <- w762 stop-if-true
          n262 = TCP Read(connection ID=w767, bytes to read=8 ("读取的字节")) -> (connection ID out=w761:refnum<k5>, data out=w765:string)  [unwired: 3 in, 1 out]
          n263 = String Subset(string=w765, length (rest)=3 ("偏移量(0)")) -> (substring=w764:string)  [unwired: 1 in]
          n264 = Equal?(x=w764, y="ACK") -> (x = y?=w762:bool)
        }
      }
    }
    n265 = Byte Array To String(unsigned byte array=w733) -> (string=w738:string)
    n266 = Byte Array To String(unsigned byte array=u8[] [3] ("无符号字节数组")) -> (string=w715:string)
    n267 = Byte Array To String(unsigned byte array=u8[] [1] ("无符号字节数组")) -> (string=w723:string)
    n268 = Byte Array To String(unsigned byte array=w707) -> (string=w717:string)
    n269 = Byte Array To String(unsigned byte array=w709) -> (string=w726:string)
    n270 = Concatenate Strings("PRExxxx" ("数据输入"), w738) -> (w736:string)
    n271 = Concatenate Strings("DIVxxx" ("数据输入"), w723, w726) -> (w725:string)
    n272 = Concatenate Strings("DIVxxx" ("数据输入"), w715, w717) -> (w700:string)
    n273 = TCP Write(connection ID=w698, data in=w736) -> (connection ID out=w747:refnum<k5>)  [unwired: 2 in, 2 out]
    n274 = while {
      tunnel: w747 -> [w807]
      tunnel: [w801] -> w742
      stop <- w802 stop-if-true
      n275 = TCP Read(connection ID=w807, bytes to read=8 ("读取的字节")) -> (connection ID out=w801:refnum<k5>, data out=w805:string)  [unwired: 3 in, 1 out]
      n276 = String Subset(string=w805, length (rest)=3 ("偏移量(0)")) -> (substring=w804:string)  [unwired: 1 in]
      n277 = Equal?(x=w804, y="ACK") -> (x = y?=w802:bool)
    }
    n278 = TCP Write(connection ID=w742, data in=w725) -> (connection ID out=w746:refnum<k5>)  [unwired: 2 in, 2 out]
    n279 = while {
      tunnel: w746 -> [w799]
      tunnel: [w793] -> w741
      stop <- w794 stop-if-true
      n280 = TCP Read(connection ID=w799, bytes to read=8 ("读取的字节")) -> (connection ID out=w793:refnum<k5>, data out=w797:string)  [unwired: 3 in, 1 out]
      n281 = String Subset(string=w797, length (rest)=3 ("偏移量(0)")) -> (substring=w796:string)  [unwired: 1 in]
      n282 = Equal?(x=w796, y="ACK") -> (x = y?=w794:bool)
    }
    n283 = Byte Array To String(unsigned byte array=u8[] [4] ("无符号字节数组")) -> (string=w711:string)
    n284 = Byte Array To String(unsigned byte array=w706) -> (string=w713:string)
    n285 = Byte Array To String(unsigned byte array=u8[] [2] ("无符号字节数组")) -> (string=w719:string)
    n286 = Byte Array To String(unsigned byte array=w708) -> (string=w721:string)
    n287 = Concatenate Strings("DIVxxx" ("数据输入"), w711, w713) -> (w704:string)
    n288 = Concatenate Strings("DIVxxx" ("数据输入"), w719, w721) -> (w705:string)
    n289 = TCP Write(connection ID=w741, data in=w705) -> (connection ID out=w745:refnum<k5>)  [unwired: 2 in, 2 out]
    n290 = while {
      tunnel: w745 -> [w791]
      tunnel: [w785] -> w740
      stop <- w786 stop-if-true
      n291 = TCP Read(connection ID=w791, bytes to read=8 ("读取的字节")) -> (connection ID out=w785:refnum<k5>, data out=w789:string)  [unwired: 3 in, 1 out]
      n292 = String Subset(string=w789, length (rest)=3 ("偏移量(0)")) -> (substring=w788:string)  [unwired: 1 in]
      n293 = Equal?(x=w788, y="ACK") -> (x = y?=w786:bool)
    }
    n294 = TCP Write(connection ID=w740, data in=w700) -> (connection ID out=w744:refnum<k5>)  [unwired: 2 in, 2 out]
    n295 = while {
      tunnel: w744 -> [w783]
      tunnel: [w777] -> w739
      stop <- w778 stop-if-true
      n296 = TCP Read(connection ID=w783, bytes to read=8 ("读取的字节")) -> (connection ID out=w777:refnum<k5>, data out=w781:string)  [unwired: 3 in, 1 out]
      n297 = String Subset(string=w781, length (rest)=3 ("偏移量(0)")) -> (substring=w780:string)  [unwired: 1 in]
      n298 = Equal?(x=w780, y="ACK") -> (x = y?=w778:bool)
    }
    n299 = TCP Write(connection ID=w739, data in=w704) -> (connection ID out=w743:refnum<k5>)  [unwired: 2 in, 2 out]
    n300 = while {
      tunnel: w743 -> [w775]
      tunnel: [w769] -> w703
      stop <- w770 stop-if-true
      n301 = TCP Read(connection ID=w775, bytes to read=8 ("读取的字节")) -> (connection ID out=w769:refnum<k5>, data out=w773:string)  [unwired: 3 in, 1 out]
      n302 = String Subset(string=w773, length (rest)=3 ("偏移量(0)")) -> (substring=w772:string)  [unwired: 1 in]
      n303 = Equal?(x=w772, y="ACK") -> (x = y?=w770:bool)
    }
    n304 = TCP Write(connection ID=w703, data in="STAxxxxx" ("数据输入")) -> (connection ID out=w701:refnum<k5>)  [unwired: 2 in, 2 out]
    n305 = while {
      tunnel: w701 -> [w856]
      tunnel: w750 -> [w855]
      tunnel: w749 -> [w828]
      tunnel: w748 -> [w808]
      stop <- w818 stop-if-true
      n306 = Get Date/Time String(want seconds? (F)=TRUE ("需要秒？(F)")) -> (date string=w826:string, time string=w823:string)  [unwired: 2 in]
      n307 = Concatenate Strings(w826, "-" ("字符串"), w823, ".bin" ("字符串")) -> (w822:string)
      n308 = Path To String(path=w828) -> (string=w839:string)
      n309 = Search and Replace String(replace all?=TRUE ("替换全部？(F)"), input string=w822, search string=":" ("搜索字符串"), replace string="-" ("替换字符串(\"\")")) -> (result string=w814:string)  [unwired: 4 in, 3 out]
      n310 = Search and Replace String(replace all?=TRUE ("替换全部？(F)"), input string=w814, search string="/" ("搜索字符串"), replace string="-" ("替换字符串(\"\")")) -> (result string=w813:string)  [unwired: 4 in, 3 out]
      n311 = Concatenate Strings(w839, "\\2振动2-" ("字符串"), w813) -> (w846:string)
      n312 = Concatenate Strings(w839, "\\2振动1-" ("字符串"), w813) -> (w845:string)
      n313 = Concatenate Strings(w839, "\\2振动4-" ("字符串"), w813) -> (w848:string)
      n314 = Concatenate Strings(w839, "\\2振动3-" ("字符串"), w813) -> (w847:string)
      n315 = Concatenate Strings(w839, "\\2转速-" ("字符串"), w813) -> (w849:string)
      n316 = String To Path(string=w846) -> (path=w843:path)
      n317 = String To Path(string=w847) -> (path=w842:path)
      n318 = String To Path(string=w845) -> (path=w844:path)
      n319 = String To Path(string=w848) -> (path=w841:path)
      n320 = String To Path(string=w849) -> (path=w840:path)
      n321 = Open/Create/Replace File(file path (use dialog)=w841, operation (0:open)=T1."open or create" ("操作(0:open)")) -> (refnum out=w830:refnum<file>)  [unwired: 4 in, 2 out]
      n322 = Open/Create/Replace File(file path (use dialog)=w843, operation (0:open)=T1."open or create" ("操作(0:open)")) -> (refnum out=w832:refnum<file>)  [unwired: 4 in, 2 out]
      n323 = Open/Create/Replace File(file path (use dialog)=w842, operation (0:open)=T1."open or create" ("操作(0:open)")) -> (refnum out=w831:refnum<file>)  [unwired: 4 in, 2 out]
      n324 = Open/Create/Replace File(file path (use dialog)=w840, operation (0:open)=T1."open or create" ("操作(0:open)")) -> (refnum out=w829:refnum<file>)  [unwired: 4 in, 2 out]
      n325 = Open/Create/Replace File(file path (use dialog)=w844, operation (0:open)=T1."open or create" ("操作(0:open)")) -> (refnum out=w833:refnum<file>)  [unwired: 4 in, 2 out]
      n326 = while {
        shift-right: [w914] -> _
        shift-left: _ -> [w913]
        shift-right: [w896] -> _
        shift-left: w856 -> [w900]
        shift-right: [w908] -> _
        shift-left: _ -> [w911]
        shift-right: [w905] -> _
        shift-left: _ -> [w906]
        shift-right: [w903] -> _
        shift-left: _ -> [w901]
        shift-right: [w892] -> _
        shift-left: w833 -> [w887]
        shift-right: [w891] -> _
        shift-left: w832 -> [w886]
        shift-right: [w890] -> _
        shift-left: w831 -> [w885]
        shift-right: [w889] -> _
        shift-left: w830 -> [w884]
        shift-right: [w888] -> _
        shift-left: w829 -> [w883]
        tunnel: w855 -> [w882]
        tunnel: [w880] -> w818
        shift-right: [w864] -> _
        shift-left: i16[] [] -> [w868]
        shift-right: [w865] -> _
        shift-left: i16[] [] -> [w869]
        shift-right: [w866] -> _
        shift-left: i16[] [] -> [w870]
        shift-right: [w867] -> _
        shift-left: i16[] [] -> [w863]
        tunnel: w808 -> [w859]
        i -> [w878]
        stop <- w879 stop-if-true
        n327 = TCP Read(connection ID=w900, bytes to read=1 ("读取的字节")) -> (connection ID out=w893:refnum<k5>, data out=w898:string)  [unwired: 3 in, 1 out]
        n328 = Equal?(x=w898, y="D") -> (x = y?=w894:bool)
        n329 = case shown="真" w894 {
          tunnel: w893 -> [w956 w977]
          tunnel: [w956 w976] -> w896
          tunnel: [0 w975] -> w895
          tunnel: [FALSE w973] -> w880
          tunnel: [w953 w972] -> w892
          tunnel: [w952 w965] -> w891
          tunnel: [w951 w964] -> w890
          tunnel: [w950 w963] -> w889
          tunnel: [w949 w971] -> w888
          tunnel: w887 -> [w953 w970]
          tunnel: w886 -> [w952 w969]
          tunnel: w885 -> [w951 w968]
          tunnel: w884 -> [w950 w967]
          tunnel: w883 -> [w949 w966]
          tunnel: w882 -> [_ w962]
          tunnel: [FALSE w961] -> w881
          tunnel: [i16[] [] w960] -> w874
          tunnel: [i16[] [] w959] -> w873
          tunnel: [i16[] [] w958] -> w872
          tunnel: [i16[] [] w957] -> w871
          frame False {
          }
          frame True {
            n330 = TCP Read(connection ID=w977, bytes to read=1 ("读取的字节")) -> (connection ID out=w974:refnum<k5>, data out=w980:string)  [unwired: 3 in, 1 out]
            n331 = Equal?(x=w980, y="A") -> (x = y?=w978:bool)
            n332 = case shown="真" w978 {
              tunnel: w974 -> [w994 w1015]
              tunnel: [w994 w1014] -> w976
              tunnel: [0 w1013] -> w975
              tunnel: [FALSE w1011] -> w973
              tunnel: [w991 w1010] -> w972
              tunnel: [w987 w1006] -> w971
              tunnel: w970 -> [w991 w1005]
              tunnel: w969 -> [w990 w1004]
              tunnel: w968 -> [w989 w1003]
              tunnel: w967 -> [w988 w1002]
              tunnel: w966 -> [w987 w1001]
              tunnel: [w990 w1009] -> w965
              tunnel: [w989 w1008] -> w964
              tunnel: [w988 w1007] -> w963
              tunnel: w962 -> [_ w1000]
              tunnel: [FALSE w999] -> w961
              tunnel: [i16[] [] w998] -> w960
              tunnel: [i16[] [] w997] -> w959
              tunnel: [i16[] [] w996] -> w958
              tunnel: [i16[] [] w995] -> w957
              frame False {
              }
              frame True {
                n333 = TCP Read(connection ID=w1015, bytes to read=1 ("读取的字节")) -> (connection ID out=w1012:refnum<k5>, data out=w1018:string)  [unwired: 3 in, 1 out]
                n334 = Equal?(x=w1018, y="T") -> (x = y?=w1016:bool)
                n335 = case shown="真" w1016 {
                  tunnel: w1012 -> [w1032 w1054]
                  tunnel: [w1032 w1051] -> w1014
                  tunnel: [0 w1053] -> w1013
                  tunnel: [FALSE w1050] -> w1011
                  tunnel: [w1025 w1042] -> w1010
                  tunnel: [w1026 w1041] -> w1009
                  tunnel: [w1027 w1040] -> w1008
                  tunnel: [w1028 w1049] -> w1007
                  tunnel: [w1029 w1048] -> w1006
                  tunnel: w1005 -> [w1025 w1047]
                  tunnel: w1004 -> [w1026 w1046]
                  tunnel: w1003 -> [w1027 w1045]
                  tunnel: w1002 -> [w1028 w1044]
                  tunnel: w1001 -> [w1029 w1043]
                  tunnel: w1000 -> [_ w1039]
                  tunnel: [FALSE w1038] -> w999
                  tunnel: [i16[] [] w1037] -> w998
                  tunnel: [i16[] [] w1036] -> w997
                  tunnel: [i16[] [] w1035] -> w996
                  tunnel: [i16[] [] w1034] -> w995
                  frame False {
                  }
                  frame True {
                    n336 = TCP Read(connection ID=w1054, bytes to read=2 ("读取的字节")) -> (connection ID out=w1052:refnum<k5>)  [unwired: 3 in, 2 out]
                    n337 = case shown="真" TRUE {
                      tunnel: w1052 -> [w1068 w1204]
                      tunnel: [0 w1195] -> w1053
                      tunnel: [w1068 w1189] -> w1051
                      tunnel: [FALSE w1190] -> w1050
                      tunnel: [w1062 w1172] -> w1049
                      tunnel: [w1061 w1171] -> w1048
                      tunnel: w1047 -> [w1065 w1178]
                      tunnel: w1046 -> [w1064 w1176]
                      tunnel: w1045 -> [w1063 w1174]
                      tunnel: w1044 -> [w1062 w1099]
                      tunnel: w1043 -> [w1061 w1170]
                      tunnel: [w1065 w1177] -> w1042
                      tunnel: [w1064 w1175] -> w1041
                      tunnel: [w1063 w1173] -> w1040
                      tunnel: w1039 -> [_ w1168]
                      tunnel: [FALSE w1166] -> w1038
                      tunnel: [i16[] [] w1098] -> w1037
                      tunnel: [i16[] [] w1097] -> w1036
                      tunnel: [i16[] [] w1096] -> w1035
                      tunnel: [i16[] [] w1095] -> w1034
                      frame False {
                      }
                      frame True {
                        n338 = TCP Read(connection ID=w1204, bytes to read=4021 ("最大值(548)")) -> (connection ID out=w1179:refnum<k5>, data out=w1188:string)  [unwired: 3 in, 1 out]
                        n339 = String To Byte Array(string=w1188) -> (unsigned byte array=w1187:u8[])
                        n340 = String Length(string=w1188) -> (length=w1195:i32)
                        n341 = Split 1D Array(array=w1187, index=1000 ("索引")) -> (first subarray=w1094:u8[], second subarray=w1091:u8[])
                        n342 = Split 1D Array(array=w1091, index=1000 ("索引")) -> (first subarray=w1090:u8[], second subarray=w1087:u8[])
                        n343 = Split 1D Array(array=w1087, index=1000 ("索引")) -> (first subarray=w1086:u8[], second subarray=w1085:u8[])
                        n344 = Split 1D Array(array=w1085, index=1000 ("索引")) -> (first subarray=w1082:u8[], second subarray=w1072:u8[])
                        n345 = Split 1D Array(array=w1072, index=2 ("索引")) -> (first subarray=w1075:u8[], second subarray=w1074:u8[])
                        n346 = Split 1D Array(array=w1074, index=2 ("索引")) -> (first subarray=w1149:u8[], second subarray=w1165:u8[])
                        n347 = Split 1D Array(array=w1165, index=2 ("索引")) -> (first subarray=w1113:u8[], second subarray=w1164:u8[])
                        n348 = Split 1D Array(array=w1164, index=2 ("索引")) -> (first subarray=w1112:u8[], second subarray=w1151:u8[])
                        n349 = Split 1D Array(array=w1151, index=2 ("索引")) -> (first subarray=w1111:u8[], second subarray=w1160:u8[])
                        n350 = Split 1D Array(array=w1160, index=2 ("索引")) -> (first subarray=w1110:u8[], second subarray=w1159:u8[])
                        n351 = Split 1D Array(array=w1159, index=2 ("索引")) -> (first subarray=w1109:u8[], second subarray=w1150:u8[])
                        n352 = Split 1D Array(array=w1150, index=2 ("索引")) -> (first subarray=w1108:u8[], second subarray=w1071:u8[])
                        n353 = Split 1D Array(array=w1071, index=5 ("索引")) -> (first subarray=w1069:u8[])  [unwired: 1 out]
                        n354 = Decimate 1D Array(w1094) -> (w1093:u8[], w1092:u8[])
                        n355 = Decimate 1D Array(w1090) -> (w1089:u8[], w1088:u8[])
                        n356 = Decimate 1D Array(w1086) -> (w1084:u8[], w1083:u8[])
                        n357 = Decimate 1D Array(w1082) -> (w1081:u8[], w1080:u8[])
                        n358 = Get Date/Time String(date format (0)=enum16{"short", "long", "abbreviated"}."short" ("日期格式(0)"), want seconds? (F)=TRUE ("需要秒？(F)")) -> (date string=w1184:string, time string=w1167:string)  [unwired: 1 in]
                        n359 = Decimate 1D Array(w1075) -> (w1077:u8[], w1076:u8[])
                        n360 = Join Numbers(hi=w1093, lo=w1092) -> ((hi.lo)=w1202:u16[])
                        n361 = Join Numbers(hi=w1089, lo=w1088) -> ((hi.lo)=w1197:u16[])
                        n362 = Join Numbers(hi=w1077, lo=w1076) -> ((hi.lo)=w1078:u16[])
                        n363 = Join Numbers(hi=w1084, lo=w1083) -> ((hi.lo)=w1198:u16[])
                        n364 = Join Numbers(hi=w1081, lo=w1080) -> ((hi.lo)=w1199:u16[])
                        n365 = Index Array(array=w1149, index=0 ("索引")) -> (element=w1144:u8)
                        n366 = Index Array(array=w1149, index=1 ("索引")) -> (element=w1146:u8)
                        n367 = String To Byte Array(string="_PSAI") -> (unsigned byte array=w1193:u8[])
                        n368 = Index Array(array=w1113, index=0 ("索引")) -> (element=w1138:u8)
                        n369 = Index Array(array=w1113, index=1 ("索引")) -> (element=w1140:u8)
                        n370 = Index Array(array=w1111, index=0 ("索引")) -> (element=w1126:u8)
                        n371 = Index Array(array=w1112, index=0 ("索引")) -> (element=w1132:u8)
                        n372 = Index Array(array=w1111, index=1 ("索引")) -> (element=w1128:u8)
                        n373 = Index Array(array=w1112, index=1 ("索引")) -> (element=w1134:u8)
                        n374 = Index Array(array=w1110, index=0 ("索引")) -> (element=w1120:u8)
                        n375 = To Word Integer(number=w1202) -> (16bit integer=w1098:i16[])
                        "?" <- w1098
                        n376 = Index Array(array=w1110, index=1 ("索引")) -> (element=w1122:u8)
                        n377 = To Word Integer(number=w1197) -> (16bit integer=w1097:i16[])
                        "?" <- w1097
                        n378 = Index Array(array=w1109, index=0 ("索引")) -> (element=w1114:u8)
                        n379 = call <vilib>:"Space Constant.vi"() -> ("String"=w1180:string)
                        n380 = Index Array(array=w1109, index=1 ("索引")) -> (element=w1116:u8)
                        n381 = To Unsigned Word Integer(number=w1078) -> (unsigned 16bit integer=w1073:u16[])
                        "?" <- w1073
                        n382 = To Word Integer(number=w1198) -> (16bit integer=w1096:i16[])
                        "?" <- w1096
                        n383 = To Word Integer(number=w1199) -> (16bit integer=w1095:i16[])
                        "?" <- w1095
                        n384 = Equal?(x=w1069, y=w1193) -> (x = y?=w1192:bool[])
                        n385 = Index Array(array=w1108, index=0 ("索引")) -> (element=→"?":u8)
                        n386 = Divide(x=w1146, y=10.0) -> (x/y=w1145:dbl)
                        n387 = Divide(x=w1140, y=10.0) -> (x/y=w1139:dbl)
                        n388 = Divide(x=w1128, y=10.0) -> (x/y=w1127:dbl)
                        n389 = Divide(x=w1134, y=10.0) -> (x/y=w1133:dbl)
                        n390 = Concatenate Strings("\r", "@@" ("字符串"), w1184, w1180, w1167, "@@" ("字符串")) -> (w1183:string)
                        "系统时间 2" <- w1183
                        n391 = Divide(x=w1122, y=10.0) -> (x/y=w1121:dbl)
                        n392 = Index Array(array=w1108, index=1 ("索引")) -> (element=→"?":u8)
                        n393 = Divide(x=w1116, y=10.0) -> (x/y=w1115:dbl)
                        n394 = And Array Elements(Boolean array=w1192) -> (logical AND=w1191:bool)
                        n395 = Add(x=w1144, y=w1145) -> (x+y=→"?":dbl)
                        n396 = Add(x=w1138, y=w1139) -> (x+y=→"?":dbl)
                        n397 = Add(x=w1126, y=w1127) -> (x+y=→"?":dbl)
                        n398 = Add(x=w1132, y=w1133) -> (x+y=→"?":dbl)
                        n399 = Add(x=w1120, y=w1121) -> (x+y=→"?":dbl)
                        n400 = Add(x=w1114, y=w1115) -> (x+y=→"?":dbl)
                        n401 = local write "系统时间 2"(w1183) -> ()
                        n402 = case shown="真" w1191 {
                          tunnel: [w1214 w1233] -> w1189
                          tunnel: [TRUE FALSE] -> w1190
                          tunnel: w1179 -> [w1212 w1233]
                          tunnel: w1098 -> [_ w1232]
                          tunnel: w1097 -> [_ w1231]
                          tunnel: w1096 -> [_ w1230]
                          tunnel: w1095 -> [_ w1229]
                          tunnel: w1073 -> [_ w1228]
                          tunnel: w1178 -> [w1210 w1226]
                          tunnel: [w1210 w1225] -> w1177
                          tunnel: w1176 -> [w1211 w1224]
                          tunnel: [w1211 w1223] -> w1175
                          tunnel: w1174 -> [w1209 w1222]
                          tunnel: [w1209 w1221] -> w1173
                          tunnel: w1099 -> [w1208 w1220]
                          tunnel: [w1208 w1219] -> w1172
                          tunnel: [w1207 w1218] -> w1171
                          tunnel: w1170 -> [w1207 w1217]
                          tunnel: w1168 -> [_ w1216]
                          tunnel: [FALSE w1215] -> w1166
                          frame False {
                            n403 = TCP Close Connection(connection ID=w1212) -> (connection ID out=w1214:refnum<k5>)  [unwired: 2 in, 1 out]
                          }
                          frame True {
                            n404 = case shown="真" w1216 {
                              tunnel: w1232 -> [_ w1286]
                              tunnel: w1231 -> [_ w1266]
                              tunnel: w1230 -> [_ w1265]
                              tunnel: w1229 -> [_ w1264]
                              tunnel: w1228 -> [_ w1263]
                              tunnel: w1226 -> [w1239 w1252]
                              tunnel: [w1239 w1243] -> w1225
                              tunnel: w1224 -> [w1238 w1251]
                              tunnel: [w1238 w1250] -> w1223
                              tunnel: w1222 -> [w1237 w1249]
                              tunnel: [w1237 w1244] -> w1221
                              tunnel: w1220 -> [w1236 w1248]
                              tunnel: [w1236 w1247] -> w1219
                              tunnel: [w1235 w1246] -> w1218
                              tunnel: w1217 -> [w1235 w1245]
                              tunnel: [FALSE w1240] -> w1215
                              frame False {
                              }
                              frame True {
                                n405 = local read "系统时间 2"() -> (w1260:string)
                                n406 = local read "系统时间 2"() -> (w1262:string)
                                n407 = local read "系统时间 2"() -> (w1254:string)
                                n408 = local read "系统时间 2"() -> (w1256:string)
                                n409 = local read "系统时间 2"() -> (w1258:string)
                                n410 = String To Byte Array(string=w1260) -> (unsigned byte array=w1259:u8[])
                                n411 = String To Byte Array(string=w1256) -> (unsigned byte array=w1255:u8[])
                                n412 = String To Byte Array(string=w1254) -> (unsigned byte array=w1253:u8[])
                                n413 = String To Byte Array(string=w1262) -> (unsigned byte array=w1261:u8[])
                                n414 = String To Byte Array(string=w1258) -> (unsigned byte array=w1257:u8[])
                                n415 = Insert Into Array(array=w1286, index=0 ("索引"), new element=w1253) -> (w1284:i16[])
                                n416 = Insert Into Array(array=w1266, index=0 ("索引"), new element=w1255) -> (w1280:i16[])
                                n417 = Insert Into Array(array=w1265, index=0 ("索引"), new element=w1257) -> (w1276:i16[])
                                n418 = Insert Into Array(array=w1264, index=0 ("索引"), new element=w1259) -> (w1272:i16[])
                                n419 = Insert Into Array(array=w1263, index=0 ("索引"), new element=w1261) -> (w1268:u16[])
                                n420 = Write to Binary File(file (use dialog)=w1252, data=w1284, 5:FALSE ("预置数组或字符串大小？(T)"), 9:T2."little-endian" ("字节顺序(0:big-endian, network order)")) -> (refnum out=w1243:refnum<file>)  [unwired: 2 in, 2 out]
                                n421 = Write to Binary File(file (use dialog)=w1251, data=w1280, 5:FALSE ("预置数组或字符串大小？(T)"), 9:T2."little-endian" ("字节顺序(0:big-endian, network order)")) -> (refnum out=w1250:refnum<file>)  [unwired: 2 in, 2 out]
                                n422 = Write to Binary File(file (use dialog)=w1249, data=w1276, 5:FALSE ("预置数组或字符串大小？(T)"), 9:T2."little-endian" ("字节顺序(0:big-endian, network order)")) -> (refnum out=w1244:refnum<file>)  [unwired: 2 in, 2 out]
                                n423 = Write to Binary File(file (use dialog)=w1248, data=w1272, 5:FALSE ("预置数组或字符串大小？(T)"), 9:T2."little-endian" ("字节顺序(0:big-endian, network order)")) -> (refnum out=w1247:refnum<file>)  [unwired: 2 in, 2 out]
                                n424 = Write to Binary File(file (use dialog)=w1245, data=w1268, 5:FALSE ("预置数组或字符串大小？(T)"), 9:T2."little-endian" ("字节顺序(0:big-endian, network order)")) -> (refnum out=w1246:refnum<file>)  [unwired: 2 in, 2 out]
                                n425 = Get File Size(file=w1243) -> (size (in bytes)=w1242:i64)  [unwired: 1 in, 2 out]
                                n426 = Greater Or Equal?(x=w1242, y=i64 60000000) -> (x >= y?=w1240:bool)
                              }
                            }
                          }
                        }
                      }
                    }
                  }
                }
              }
            }
          }
        }
        n427 = Divide(x=u8 187, y=w859) -> (x/y=w857:dbl)
        n428 = Round Toward -Infinity(1:w857) -> (0:w861:dbl)
        n429 = Multiply(x=w861, y=500.0) -> (x*y=w860:dbl)
        n430 = Quotient & Remainder(x=w878, y=w861) -> (x-y*floor(x/y)=w877:dbl)  [unwired: 1 out]
        n431 = Equal?(x=w877, y=0) -> (x = y?=w875:bool)
        n432 = case shown="真" w875 {
          tunnel: w874 -> [w918 w943]
          tunnel: w873 -> [w917 w942]
          tunnel: w872 -> [w916 w941]
          tunnel: w871 -> [w915 w940]
          tunnel: [w926 w943] -> w864
          tunnel: [w925 w942] -> w865
          tunnel: [w924 w941] -> w866
          tunnel: [w923 w940] -> w867
          tunnel: w863 -> [w922 w936]
          tunnel: w870 -> [w921 w939]
          tunnel: w869 -> [w920 w937]
          tunnel: w868 -> [w919 w938]
          tunnel: w860 -> [_ w931]
          frame False {
            n433 = Array Size(array=w921) -> (size(s)=w928:i32)
            n434 = Array Size(array=w922) -> (size(s)=w927:i32)
            n435 = Array Size(array=w919) -> (size(s)=w930:i32)
            n436 = Array Size(array=w920) -> (size(s)=w929:i32)
            n437 = Insert Into Array(array=w921, index=w928, new element=w916) -> (w924:i16[])
            n438 = Insert Into Array(array=w922, index=w927, new element=w915) -> (w923:i16[])
            n439 = Insert Into Array(array=w919, index=w930, new element=w918) -> (w926:i16[])
            n440 = Insert Into Array(array=w920, index=w929, new element=w917) -> (w925:i16[])
          }
          frame True {
            n441 = call <vilib>:"Amplitude and Phase Spectrum.vi"("dt"=w931, "Signal (V)"=w937) -> ("Amp Spectrum Mag (Vrms)"=→"?":dbl[])  [unwired: 1 in, 2 out]
            n442 = call <vilib>:"Amplitude and Phase Spectrum.vi"("dt"=w931, "Signal (V)"=w936) -> ("Amp Spectrum Mag (Vrms)"=→"?":dbl[])  [unwired: 1 in, 2 out]
            n443 = call <vilib>:"Amplitude and Phase Spectrum.vi"("dt"=w931, "Signal (V)"=w938) -> ("Amp Spectrum Mag (Vrms)"=→"?":dbl[])  [unwired: 1 in, 2 out]
            n444 = call <vilib>:"Amplitude and Phase Spectrum.vi"("dt"=w931, "Signal (V)"=w939) -> ("Amp Spectrum Mag (Vrms)"=→"?":dbl[])  [unwired: 1 in, 2 out]
          }
        }
        n445 = Add(x=w913, y=w895) -> (x+y=w914:i32)
        "收包 2" <- w914
        n446 = Tick Count (ms)() -> (millisecond timer value=w905:u32)
        n447 = Subtract(x=w905, y=w906) -> (x-y=w904:u32)
        n448 = Subtract(x=w914, y=w913) -> (x-y=w912:i32)
        n449 = Add(x=w912, y=w911) -> (x+y=w907:i32)
        n450 = Add(x=w901, y=w904) -> (x+y=w902:u32)
        n451 = Greater Or Equal?(x=w907, y=1000000) -> (x >= y?=w909:bool)
        n452 = Or(x=w881, y=w880) -> (x .or. y?=w879:bool)
        n453 = case shown="真" w909 {
          tunnel: [w1289 0] -> w908
          tunnel: w907 -> [w1289 w1292]
          tunnel: [w1288 u32 0] -> w903
          tunnel: w902 -> [w1288 w1293]
          frame False {
          }
          frame True {
            n454 = Divide(x=w1292, y=w1293) -> (x/y=→"KB/s 2":dbl)
          }
        }
      }
    }
  }
  n455 = while {
    tunnel: w7 -> [w1347]
    tunnel: w8 -> [w1346]
    tunnel: w5 -> [w1332]
    tunnel: w6 -> [w1345]
    stop <- FALSE stop-if-true
    n456 = Split 1D Array(array=w1332, index=1 ("索引")) -> (first subarray=w1330:u8[], second subarray=w1326:u8[])
    n457 = Split 1D Array(array=w1326, index=1 ("索引")) -> (first subarray=w1306:u8[], second subarray=w1325:u8[])
    n458 = Split 1D Array(array=w1325, index=1 ("索引")) -> (first subarray=w1305:u8[], second subarray=w1324:u8[])
    n459 = Split 1D Array(array=w1324, index=1 ("索引")) -> (first subarray=w1304:u8[], second subarray=w1303:u8[])
    n460 = flat-sequence {
      tunnel: [w1350] -> w1296
      tunnel: w1296 -> [w1355]
      tunnel: [w1353] -> w1295
      frame #0 {
        n461 = Wait (ms)(milliseconds to wait=u32 1000 ("毫秒倍数")) -> ()  [unwired: 1 out]
      }
      frame #1 {
        n462 = TCP Open Connection(address="192.168.1.17" ("名称"), remote port or service name=u16 3857 ("端口")) -> (connection ID=w1350:refnum<k5>)  [unwired: 3 in, 1 out]
      }
      frame #2 {
        n463 = TCP Write(connection ID=w1355, data in="INTxxxxx" ("数据输入")) -> (connection ID out=w1354:refnum<k5>)  [unwired: 2 in, 2 out]
        n464 = while {
          tunnel: w1354 -> [w1364]
          tunnel: [w1358] -> w1353
          stop <- w1359 stop-if-true
          n465 = TCP Read(connection ID=w1364, bytes to read=8 ("读取的字节")) -> (connection ID out=w1358:refnum<k5>, data out=w1362:string)  [unwired: 3 in, 1 out]
          n466 = String Subset(string=w1362, length (rest)=3 ("偏移量(0)")) -> (substring=w1361:string)  [unwired: 1 in]
          n467 = Equal?(x=w1361, y="ACK") -> (x = y?=w1359:bool)
        }
      }
    }
    n468 = Byte Array To String(unsigned byte array=w1330) -> (string=w1335:string)
    n469 = Byte Array To String(unsigned byte array=u8[] [3] ("无符号字节数组")) -> (string=w1312:string)
    n470 = Byte Array To String(unsigned byte array=u8[] [1] ("无符号字节数组")) -> (string=w1320:string)
    n471 = Byte Array To String(unsigned byte array=w1304) -> (string=w1314:string)
    n472 = Byte Array To String(unsigned byte array=w1306) -> (string=w1323:string)
    n473 = Concatenate Strings("PRExxxx" ("数据输入"), w1335) -> (w1333:string)
    n474 = Concatenate Strings("DIVxxx" ("数据输入"), w1320, w1323) -> (w1322:string)
    n475 = Concatenate Strings("DIVxxx" ("数据输入"), w1312, w1314) -> (w1297:string)
    n476 = TCP Write(connection ID=w1295, data in=w1333) -> (connection ID out=w1344:refnum<k5>)  [unwired: 2 in, 2 out]
    n477 = while {
      tunnel: w1344 -> [w1404]
      tunnel: [w1398] -> w1339
      stop <- w1399 stop-if-true
      n478 = TCP Read(connection ID=w1404, bytes to read=8 ("读取的字节")) -> (connection ID out=w1398:refnum<k5>, data out=w1402:string)  [unwired: 3 in, 1 out]
      n479 = String Subset(string=w1402, length (rest)=3 ("偏移量(0)")) -> (substring=w1401:string)  [unwired: 1 in]
      n480 = Equal?(x=w1401, y="ACK") -> (x = y?=w1399:bool)
    }
    n481 = TCP Write(connection ID=w1339, data in=w1322) -> (connection ID out=w1343:refnum<k5>)  [unwired: 2 in, 2 out]
    n482 = while {
      tunnel: w1343 -> [w1396]
      tunnel: [w1390] -> w1338
      stop <- w1391 stop-if-true
      n483 = TCP Read(connection ID=w1396, bytes to read=8 ("读取的字节")) -> (connection ID out=w1390:refnum<k5>, data out=w1394:string)  [unwired: 3 in, 1 out]
      n484 = String Subset(string=w1394, length (rest)=3 ("偏移量(0)")) -> (substring=w1393:string)  [unwired: 1 in]
      n485 = Equal?(x=w1393, y="ACK") -> (x = y?=w1391:bool)
    }
    n486 = Byte Array To String(unsigned byte array=u8[] [4] ("无符号字节数组")) -> (string=w1308:string)
    n487 = Byte Array To String(unsigned byte array=w1303) -> (string=w1310:string)
    n488 = Byte Array To String(unsigned byte array=u8[] [2] ("无符号字节数组")) -> (string=w1316:string)
    n489 = Byte Array To String(unsigned byte array=w1305) -> (string=w1318:string)
    n490 = Concatenate Strings("DIVxxx" ("数据输入"), w1308, w1310) -> (w1301:string)
    n491 = Concatenate Strings("DIVxxx" ("数据输入"), w1316, w1318) -> (w1302:string)
    n492 = TCP Write(connection ID=w1338, data in=w1302) -> (connection ID out=w1342:refnum<k5>)  [unwired: 2 in, 2 out]
    n493 = while {
      tunnel: w1342 -> [w1388]
      tunnel: [w1382] -> w1337
      stop <- w1383 stop-if-true
      n494 = TCP Read(connection ID=w1388, bytes to read=8 ("读取的字节")) -> (connection ID out=w1382:refnum<k5>, data out=w1386:string)  [unwired: 3 in, 1 out]
      n495 = String Subset(string=w1386, length (rest)=3 ("偏移量(0)")) -> (substring=w1385:string)  [unwired: 1 in]
      n496 = Equal?(x=w1385, y="ACK") -> (x = y?=w1383:bool)
    }
    n497 = TCP Write(connection ID=w1337, data in=w1297) -> (connection ID out=w1341:refnum<k5>)  [unwired: 2 in, 2 out]
    n498 = while {
      tunnel: w1341 -> [w1380]
      tunnel: [w1374] -> w1336
      stop <- w1375 stop-if-true
      n499 = TCP Read(connection ID=w1380, bytes to read=8 ("读取的字节")) -> (connection ID out=w1374:refnum<k5>, data out=w1378:string)  [unwired: 3 in, 1 out]
      n500 = String Subset(string=w1378, length (rest)=3 ("偏移量(0)")) -> (substring=w1377:string)  [unwired: 1 in]
      n501 = Equal?(x=w1377, y="ACK") -> (x = y?=w1375:bool)
    }
    n502 = TCP Write(connection ID=w1336, data in=w1301) -> (connection ID out=w1340:refnum<k5>)  [unwired: 2 in, 2 out]
    n503 = while {
      tunnel: w1340 -> [w1372]
      tunnel: [w1366] -> w1300
      stop <- w1367 stop-if-true
      n504 = TCP Read(connection ID=w1372, bytes to read=8 ("读取的字节")) -> (connection ID out=w1366:refnum<k5>, data out=w1370:string)  [unwired: 3 in, 1 out]
      n505 = String Subset(string=w1370, length (rest)=3 ("偏移量(0)")) -> (substring=w1369:string)  [unwired: 1 in]
      n506 = Equal?(x=w1369, y="ACK") -> (x = y?=w1367:bool)
    }
    n507 = TCP Write(connection ID=w1300, data in="STAxxxxx" ("数据输入")) -> (connection ID out=w1298:refnum<k5>)  [unwired: 2 in, 2 out]
    n508 = while {
      tunnel: w1298 -> [w1453]
      tunnel: w1347 -> [w1452]
      tunnel: w1346 -> [w1425]
      tunnel: w1345 -> [w1405]
      stop <- w1415 stop-if-true
      n509 = Get Date/Time String(want seconds? (F)=TRUE ("需要秒？(F)")) -> (date string=w1423:string, time string=w1420:string)  [unwired: 2 in]
      n510 = Concatenate Strings(w1423, "-" ("字符串"), w1420, ".bin" ("字符串")) -> (w1419:string)
      n511 = Path To String(path=w1425) -> (string=w1436:string)
      n512 = Search and Replace String(replace all?=TRUE ("替换全部？(F)"), input string=w1419, search string=":" ("搜索字符串"), replace string="-" ("替换字符串(\"\")")) -> (result string=w1411:string)  [unwired: 4 in, 3 out]
      n513 = Search and Replace String(replace all?=TRUE ("替换全部？(F)"), input string=w1411, search string="/" ("搜索字符串"), replace string="-" ("替换字符串(\"\")")) -> (result string=w1410:string)  [unwired: 4 in, 3 out]
      n514 = Concatenate Strings(w1436, "\\2振动2-" ("字符串"), w1410) -> (w1443:string)
      n515 = Concatenate Strings(w1436, "\\2振动1-" ("字符串"), w1410) -> (w1442:string)
      n516 = Concatenate Strings(w1436, "\\2振动4-" ("字符串"), w1410) -> (w1445:string)
      n517 = Concatenate Strings(w1436, "\\2振动3-" ("字符串"), w1410) -> (w1444:string)
      n518 = Concatenate Strings(w1436, "\\2转速-" ("字符串"), w1410) -> (w1446:string)
      n519 = String To Path(string=w1443) -> (path=w1440:path)
      n520 = String To Path(string=w1444) -> (path=w1439:path)
      n521 = String To Path(string=w1442) -> (path=w1441:path)
      n522 = String To Path(string=w1445) -> (path=w1438:path)
      n523 = String To Path(string=w1446) -> (path=w1437:path)
      n524 = Open/Create/Replace File(file path (use dialog)=w1438, operation (0:open)=T1."open or create" ("操作(0:open)")) -> (refnum out=w1427:refnum<file>)  [unwired: 4 in, 2 out]
      n525 = Open/Create/Replace File(file path (use dialog)=w1440, operation (0:open)=T1."open or create" ("操作(0:open)")) -> (refnum out=w1429:refnum<file>)  [unwired: 4 in, 2 out]
      n526 = Open/Create/Replace File(file path (use dialog)=w1439, operation (0:open)=T1."open or create" ("操作(0:open)")) -> (refnum out=w1428:refnum<file>)  [unwired: 4 in, 2 out]
      n527 = Open/Create/Replace File(file path (use dialog)=w1437, operation (0:open)=T1."open or create" ("操作(0:open)")) -> (refnum out=w1426:refnum<file>)  [unwired: 4 in, 2 out]
      n528 = Open/Create/Replace File(file path (use dialog)=w1441, operation (0:open)=T1."open or create" ("操作(0:open)")) -> (refnum out=w1430:refnum<file>)  [unwired: 4 in, 2 out]
      n529 = while {
        shift-right: [w1511] -> _
        shift-left: _ -> [w1510]
        shift-right: [w1493] -> _
        shift-left: w1453 -> [w1497]
        shift-right: [w1505] -> _
        shift-left: _ -> [w1508]
        shift-right: [w1502] -> _
        shift-left: _ -> [w1503]
        shift-right: [w1500] -> _
        shift-left: _ -> [w1498]
        shift-right: [w1489] -> _
        shift-left: w1430 -> [w1484]
        shift-right: [w1488] -> _
        shift-left: w1429 -> [w1483]
        shift-right: [w1487] -> _
        shift-left: w1428 -> [w1482]
        shift-right: [w1486] -> _
        shift-left: w1427 -> [w1481]
        shift-right: [w1485] -> _
        shift-left: w1426 -> [w1480]
        tunnel: w1452 -> [w1479]
        tunnel: [w1477] -> w1415
        shift-right: [w1461] -> _
        shift-left: i16[] [] -> [w1465]
        shift-right: [w1462] -> _
        shift-left: i16[] [] -> [w1466]
        shift-right: [w1463] -> _
        shift-left: i16[] [] -> [w1467]
        shift-right: [w1464] -> _
        shift-left: i16[] [] -> [w1460]
        tunnel: w1405 -> [w1456]
        i -> [w1475]
        stop <- w1476 stop-if-true
        n530 = TCP Read(connection ID=w1497, bytes to read=1 ("读取的字节")) -> (connection ID out=w1490:refnum<k5>, data out=w1495:string)  [unwired: 3 in, 1 out]
        n531 = Equal?(x=w1495, y="D") -> (x = y?=w1491:bool)
        n532 = case shown="真" w1491 {
          tunnel: w1490 -> [w1553 w1574]
          tunnel: [w1553 w1573] -> w1493
          tunnel: [0 w1572] -> w1492
          tunnel: [FALSE w1570] -> w1477
          tunnel: [w1550 w1569] -> w1489
          tunnel: [w1549 w1562] -> w1488
          tunnel: [w1548 w1561] -> w1487
          tunnel: [w1547 w1560] -> w1486
          tunnel: [w1546 w1568] -> w1485
          tunnel: w1484 -> [w1550 w1567]
          tunnel: w1483 -> [w1549 w1566]
          tunnel: w1482 -> [w1548 w1565]
          tunnel: w1481 -> [w1547 w1564]
          tunnel: w1480 -> [w1546 w1563]
          tunnel: w1479 -> [_ w1559]
          tunnel: [FALSE w1558] -> w1478
          tunnel: [i16[] [] w1557] -> w1471
          tunnel: [i16[] [] w1556] -> w1470
          tunnel: [i16[] [] w1555] -> w1469
          tunnel: [i16[] [] w1554] -> w1468
          frame False {
          }
          frame True {
            n533 = TCP Read(connection ID=w1574, bytes to read=1 ("读取的字节")) -> (connection ID out=w1571:refnum<k5>, data out=w1577:string)  [unwired: 3 in, 1 out]
            n534 = Equal?(x=w1577, y="A") -> (x = y?=w1575:bool)
            n535 = case shown="真" w1575 {
              tunnel: w1571 -> [w1591 w1612]
              tunnel: [w1591 w1611] -> w1573
              tunnel: [0 w1610] -> w1572
              tunnel: [FALSE w1608] -> w1570
              tunnel: [w1588 w1607] -> w1569
              tunnel: [w1584 w1603] -> w1568
              tunnel: w1567 -> [w1588 w1602]
              tunnel: w1566 -> [w1587 w1601]
              tunnel: w1565 -> [w1586 w1600]
              tunnel: w1564 -> [w1585 w1599]
              tunnel: w1563 -> [w1584 w1598]
              tunnel: [w1587 w1606] -> w1562
              tunnel: [w1586 w1605] -> w1561
              tunnel: [w1585 w1604] -> w1560
              tunnel: w1559 -> [_ w1597]
              tunnel: [FALSE w1596] -> w1558
              tunnel: [i16[] [] w1595] -> w1557
              tunnel: [i16[] [] w1594] -> w1556
              tunnel: [i16[] [] w1593] -> w1555
              tunnel: [i16[] [] w1592] -> w1554
              frame False {
              }
              frame True {
                n536 = TCP Read(connection ID=w1612, bytes to read=1 ("读取的字节")) -> (connection ID out=w1609:refnum<k5>, data out=w1615:string)  [unwired: 3 in, 1 out]
                n537 = Equal?(x=w1615, y="T") -> (x = y?=w1613:bool)
                n538 = case shown="真" w1613 {
                  tunnel: w1609 -> [w1629 w1651]
                  tunnel: [w1629 w1648] -> w1611
                  tunnel: [0 w1650] -> w1610
                  tunnel: [FALSE w1647] -> w1608
                  tunnel: [w1622 w1639] -> w1607
                  tunnel: [w1623 w1638] -> w1606
                  tunnel: [w1624 w1637] -> w1605
                  tunnel: [w1625 w1646] -> w1604
                  tunnel: [w1626 w1645] -> w1603
                  tunnel: w1602 -> [w1622 w1644]
                  tunnel: w1601 -> [w1623 w1643]
                  tunnel: w1600 -> [w1624 w1642]
                  tunnel: w1599 -> [w1625 w1641]
                  tunnel: w1598 -> [w1626 w1640]
                  tunnel: w1597 -> [_ w1636]
                  tunnel: [FALSE w1635] -> w1596
                  tunnel: [i16[] [] w1634] -> w1595
                  tunnel: [i16[] [] w1633] -> w1594
                  tunnel: [i16[] [] w1632] -> w1593
                  tunnel: [i16[] [] w1631] -> w1592
                  frame False {
                  }
                  frame True {
                    n539 = TCP Read(connection ID=w1651, bytes to read=2 ("读取的字节")) -> (connection ID out=w1649:refnum<k5>)  [unwired: 3 in, 2 out]
                    n540 = case shown="真" TRUE {
                      tunnel: w1649 -> [w1665 w1801]
                      tunnel: [0 w1792] -> w1650
                      tunnel: [w1665 w1786] -> w1648
                      tunnel: [FALSE w1787] -> w1647
                      tunnel: [w1659 w1769] -> w1646
                      tunnel: [w1658 w1768] -> w1645
                      tunnel: w1644 -> [w1662 w1775]
                      tunnel: w1643 -> [w1661 w1773]
                      tunnel: w1642 -> [w1660 w1771]
                      tunnel: w1641 -> [w1659 w1696]
                      tunnel: w1640 -> [w1658 w1767]
                      tunnel: [w1662 w1774] -> w1639
                      tunnel: [w1661 w1772] -> w1638
                      tunnel: [w1660 w1770] -> w1637
                      tunnel: w1636 -> [_ w1765]
                      tunnel: [FALSE w1763] -> w1635
                      tunnel: [i16[] [] w1695] -> w1634
                      tunnel: [i16[] [] w1694] -> w1633
                      tunnel: [i16[] [] w1693] -> w1632
                      tunnel: [i16[] [] w1692] -> w1631
                      frame False {
                      }
                      frame True {
                        n541 = TCP Read(connection ID=w1801, bytes to read=4021 ("最大值(548)")) -> (connection ID out=w1776:refnum<k5>, data out=w1785:string)  [unwired: 3 in, 1 out]
                        n542 = String To Byte Array(string=w1785) -> (unsigned byte array=w1784:u8[])
                        n543 = String Length(string=w1785) -> (length=w1792:i32)
                        n544 = Split 1D Array(array=w1784, index=1000 ("索引")) -> (first subarray=w1691:u8[], second subarray=w1688:u8[])
                        n545 = Split 1D Array(array=w1688, index=1000 ("索引")) -> (first subarray=w1687:u8[], second subarray=w1684:u8[])
                        n546 = Split 1D Array(array=w1684, index=1000 ("索引")) -> (first subarray=w1683:u8[], second subarray=w1682:u8[])
                        n547 = Split 1D Array(array=w1682, index=1000 ("索引")) -> (first subarray=w1679:u8[], second subarray=w1671:u8[])
                        n548 = Split 1D Array(array=w1671, index=2 ("索引")) -> (first subarray=w1672:u8[], second subarray=w1669:u8[])
                        n549 = Split 1D Array(array=w1669, index=2 ("索引")) -> (first subarray=w1746:u8[], second subarray=w1762:u8[])
                        n550 = Split 1D Array(array=w1762, index=2 ("索引")) -> (first subarray=w1710:u8[], second subarray=w1761:u8[])
                        n551 = Split 1D Array(array=w1761, index=2 ("索引")) -> (first subarray=w1709:u8[], second subarray=w1748:u8[])
                        n552 = Split 1D Array(array=w1748, index=2 ("索引")) -> (first subarray=w1708:u8[], second subarray=w1757:u8[])
                        n553 = Split 1D Array(array=w1757, index=2 ("索引")) -> (first subarray=w1707:u8[], second subarray=w1756:u8[])
                        n554 = Split 1D Array(array=w1756, index=2 ("索引")) -> (first subarray=w1706:u8[], second subarray=w1747:u8[])
                        n555 = Split 1D Array(array=w1747, index=2 ("索引")) -> (first subarray=w1705:u8[], second subarray=w1668:u8[])
                        n556 = Split 1D Array(array=w1668, index=5 ("索引")) -> (first subarray=w1666:u8[])  [unwired: 1 out]
                        n557 = Decimate 1D Array(w1691) -> (w1690:u8[], w1689:u8[])
                        n558 = Decimate 1D Array(w1687) -> (w1686:u8[], w1685:u8[])
                        n559 = Decimate 1D Array(w1683) -> (w1681:u8[], w1680:u8[])
                        n560 = Decimate 1D Array(w1679) -> (w1678:u8[], w1677:u8[])
                        n561 = Decimate 1D Array(w1672) -> (w1674:u8[], w1673:u8[])
                        n562 = Get Date/Time String(date format (0)=enum16{"short", "long", "abbreviated"}."short" ("日期格式(0)"), want seconds? (F)=TRUE ("需要秒？(F)")) -> (date string=w1781:string, time string=w1764:string)  [unwired: 1 in]
                        n563 = Join Numbers(hi=w1674, lo=w1673) -> ((hi.lo)=w1675:u16[])
                        n564 = Join Numbers(hi=w1690, lo=w1689) -> ((hi.lo)=w1799:u16[])
                        n565 = Join Numbers(hi=w1686, lo=w1685) -> ((hi.lo)=w1794:u16[])
                        n566 = Join Numbers(hi=w1681, lo=w1680) -> ((hi.lo)=w1795:u16[])
                        n567 = Join Numbers(hi=w1678, lo=w1677) -> ((hi.lo)=w1796:u16[])
                        n568 = Index Array(array=w1746, index=0 ("索引")) -> (element=w1741:u8)
                        n569 = Index Array(array=w1746, index=1 ("索引")) -> (element=w1743:u8)
                        n570 = String To Byte Array(string="_PSAI") -> (unsigned byte array=w1790:u8[])
                        n571 = Index Array(array=w1710, index=0 ("索引")) -> (element=w1735:u8)
                        n572 = Index Array(array=w1710, index=1 ("索引")) -> (element=w1737:u8)
                        n573 = Index Array(array=w1708, index=0 ("索引")) -> (element=w1723:u8)
                        n574 = Index Array(array=w1709, index=0 ("索引")) -> (element=w1729:u8)
                        n575 = To Unsigned Word Integer(number=w1675) -> (unsigned 16bit integer=w1670:u16[])
                        "?" <- w1670
                        n576 = Index Array(array=w1708, index=1 ("索引")) -> (element=w1725:u8)
                        n577 = Index Array(array=w1709, index=1 ("索引")) -> (element=w1731:u8)
                        n578 = Index Array(array=w1707, index=0 ("索引")) -> (element=w1717:u8)
                        n579 = To Word Integer(number=w1799) -> (16bit integer=w1695:i16[])
                        "?" <- w1695
                        n580 = Index Array(array=w1707, index=1 ("索引")) -> (element=w1719:u8)
                        n581 = To Word Integer(number=w1794) -> (16bit integer=w1694:i16[])
                        "?" <- w1694
                        n582 = Index Array(array=w1706, index=0 ("索引")) -> (element=w1711:u8)
                        n583 = call <vilib>:"Space Constant.vi"() -> ("String"=w1777:string)
                        n584 = Index Array(array=w1706, index=1 ("索引")) -> (element=w1713:u8)
                        n585 = To Word Integer(number=w1795) -> (16bit integer=w1693:i16[])
                        "?" <- w1693
                        n586 = To Word Integer(number=w1796) -> (16bit integer=w1692:i16[])
                        "?" <- w1692
                        n587 = Equal?(x=w1666, y=w1790) -> (x = y?=w1789:bool[])
                        n588 = Index Array(array=w1705, index=0 ("索引")) -> (element=→"?":u8)
                        n589 = Divide(x=w1743, y=10.0) -> (x/y=w1742:dbl)
                        n590 = Divide(x=w1737, y=10.0) -> (x/y=w1736:dbl)
                        n591 = Divide(x=w1725, y=10.0) -> (x/y=w1724:dbl)
                        n592 = Divide(x=w1731, y=10.0) -> (x/y=w1730:dbl)
                        n593 = Concatenate Strings("\r", "@@" ("字符串"), w1781, w1777, w1764, "@@" ("字符串")) -> (w1780:string)
                        "系统时间 3" <- w1780
                        n594 = Divide(x=w1719, y=10.0) -> (x/y=w1718:dbl)
                        n595 = Index Array(array=w1705, index=1 ("索引")) -> (element=→"?":u8)
                        n596 = Divide(x=w1713, y=10.0) -> (x/y=w1712:dbl)
                        n597 = And Array Elements(Boolean array=w1789) -> (logical AND=w1788:bool)
                        n598 = Add(x=w1741, y=w1742) -> (x+y=→"?":dbl)
                        n599 = Add(x=w1735, y=w1736) -> (x+y=→"?":dbl)
                        n600 = Add(x=w1723, y=w1724) -> (x+y=→"?":dbl)
                        n601 = Add(x=w1729, y=w1730) -> (x+y=→"?":dbl)
                        n602 = Add(x=w1717, y=w1718) -> (x+y=→"?":dbl)
                        n603 = Add(x=w1711, y=w1712) -> (x+y=→"?":dbl)
                        n604 = local write "系统时间 3"(w1780) -> ()
                        n605 = case shown="真" w1788 {
                          tunnel: [w1811 w1830] -> w1786
                          tunnel: [TRUE FALSE] -> w1787
                          tunnel: w1776 -> [w1809 w1830]
                          tunnel: w1695 -> [_ w1829]
                          tunnel: w1694 -> [_ w1828]
                          tunnel: w1693 -> [_ w1827]
                          tunnel: w1692 -> [_ w1826]
                          tunnel: w1670 -> [_ w1825]
                          tunnel: w1775 -> [w1807 w1823]
                          tunnel: [w1807 w1822] -> w1774
                          tunnel: w1773 -> [w1808 w1821]
                          tunnel: [w1808 w1820] -> w1772
                          tunnel: w1771 -> [w1806 w1819]
                          tunnel: [w1806 w1818] -> w1770
                          tunnel: w1696 -> [w1805 w1817]
                          tunnel: [w1805 w1816] -> w1769
                          tunnel: [w1804 w1815] -> w1768
                          tunnel: w1767 -> [w1804 w1814]
                          tunnel: w1765 -> [_ w1813]
                          tunnel: [FALSE w1812] -> w1763
                          frame False {
                            n606 = TCP Close Connection(connection ID=w1809) -> (connection ID out=w1811:refnum<k5>)  [unwired: 2 in, 1 out]
                          }
                          frame True {
                            n607 = case shown="真" w1813 {
                              tunnel: w1829 -> [_ w1883]
                              tunnel: w1828 -> [_ w1863]
                              tunnel: w1827 -> [_ w1862]
                              tunnel: w1826 -> [_ w1861]
                              tunnel: w1825 -> [_ w1860]
                              tunnel: w1823 -> [w1836 w1849]
                              tunnel: [w1836 w1840] -> w1822
                              tunnel: w1821 -> [w1835 w1848]
                              tunnel: [w1835 w1847] -> w1820
                              tunnel: w1819 -> [w1834 w1846]
                              tunnel: [w1834 w1841] -> w1818
                              tunnel: w1817 -> [w1833 w1845]
                              tunnel: [w1833 w1844] -> w1816
                              tunnel: [w1832 w1843] -> w1815
                              tunnel: w1814 -> [w1832 w1842]
                              tunnel: [FALSE w1837] -> w1812
                              frame False {
                              }
                              frame True {
                                n608 = local read "系统时间 3"() -> (w1857:string)
                                n609 = local read "系统时间 3"() -> (w1859:string)
                                n610 = local read "系统时间 3"() -> (w1851:string)
                                n611 = local read "系统时间 3"() -> (w1853:string)
                                n612 = local read "系统时间 3"() -> (w1855:string)
                                n613 = String To Byte Array(string=w1857) -> (unsigned byte array=w1856:u8[])
                                n614 = String To Byte Array(string=w1853) -> (unsigned byte array=w1852:u8[])
                                n615 = String To Byte Array(string=w1851) -> (unsigned byte array=w1850:u8[])
                                n616 = String To Byte Array(string=w1859) -> (unsigned byte array=w1858:u8[])
                                n617 = String To Byte Array(string=w1855) -> (unsigned byte array=w1854:u8[])
                                n618 = Insert Into Array(array=w1883, index=0 ("索引"), new element=w1850) -> (w1881:i16[])
                                n619 = Insert Into Array(array=w1863, index=0 ("索引"), new element=w1852) -> (w1877:i16[])
                                n620 = Insert Into Array(array=w1862, index=0 ("索引"), new element=w1854) -> (w1873:i16[])
                                n621 = Insert Into Array(array=w1861, index=0 ("索引"), new element=w1856) -> (w1869:i16[])
                                n622 = Insert Into Array(array=w1860, index=0 ("索引"), new element=w1858) -> (w1865:u16[])
                                n623 = Write to Binary File(file (use dialog)=w1849, data=w1881, 5:FALSE ("预置数组或字符串大小？(T)"), 9:T2."little-endian" ("字节顺序(0:big-endian, network order)")) -> (refnum out=w1840:refnum<file>)  [unwired: 2 in, 2 out]
                                n624 = Write to Binary File(file (use dialog)=w1848, data=w1877, 5:FALSE ("预置数组或字符串大小？(T)"), 9:T2."little-endian" ("字节顺序(0:big-endian, network order)")) -> (refnum out=w1847:refnum<file>)  [unwired: 2 in, 2 out]
                                n625 = Write to Binary File(file (use dialog)=w1846, data=w1873, 5:FALSE ("预置数组或字符串大小？(T)"), 9:T2."little-endian" ("字节顺序(0:big-endian, network order)")) -> (refnum out=w1841:refnum<file>)  [unwired: 2 in, 2 out]
                                n626 = Write to Binary File(file (use dialog)=w1845, data=w1869, 5:FALSE ("预置数组或字符串大小？(T)"), 9:T2."little-endian" ("字节顺序(0:big-endian, network order)")) -> (refnum out=w1844:refnum<file>)  [unwired: 2 in, 2 out]
                                n627 = Write to Binary File(file (use dialog)=w1842, data=w1865, 5:FALSE ("预置数组或字符串大小？(T)"), 9:T2."little-endian" ("字节顺序(0:big-endian, network order)")) -> (refnum out=w1843:refnum<file>)  [unwired: 2 in, 2 out]
                                n628 = Get File Size(file=w1840) -> (size (in bytes)=w1839:i64)  [unwired: 1 in, 2 out]
                                n629 = Greater Or Equal?(x=w1839, y=i64 60000000) -> (x >= y?=w1837:bool)
                              }
                            }
                          }
                        }
                      }
                    }
                  }
                }
              }
            }
          }
        }
        n630 = Divide(x=u8 187, y=w1456) -> (x/y=w1454:dbl)
        n631 = Round Toward -Infinity(1:w1454) -> (0:w1458:dbl)
        n632 = Multiply(x=w1458, y=500.0) -> (x*y=w1457:dbl)
        n633 = Quotient & Remainder(x=w1475, y=w1458) -> (x-y*floor(x/y)=w1474:dbl)  [unwired: 1 out]
        n634 = Equal?(x=w1474, y=0) -> (x = y?=w1472:bool)
        n635 = case shown="假" w1472 {
          tunnel: w1471 -> [w1515 w1540]
          tunnel: w1470 -> [w1514 w1539]
          tunnel: w1469 -> [w1513 w1538]
          tunnel: w1468 -> [w1512 w1537]
          tunnel: [w1523 w1540] -> w1461
          tunnel: [w1522 w1539] -> w1462
          tunnel: [w1521 w1538] -> w1463
          tunnel: [w1520 w1537] -> w1464
          tunnel: w1460 -> [w1519 w1533]
          tunnel: w1467 -> [w1518 w1536]
          tunnel: w1466 -> [w1517 w1534]
          tunnel: w1465 -> [w1516 w1535]
          tunnel: w1457 -> [_ w1528]
          frame False {
            n636 = Array Size(array=w1518) -> (size(s)=w1525:i32)
            n637 = Array Size(array=w1519) -> (size(s)=w1524:i32)
            n638 = Array Size(array=w1516) -> (size(s)=w1527:i32)
            n639 = Array Size(array=w1517) -> (size(s)=w1526:i32)
            n640 = Insert Into Array(array=w1518, index=w1525, new element=w1513) -> (w1521:i16[])
            n641 = Insert Into Array(array=w1519, index=w1524, new element=w1512) -> (w1520:i16[])
            n642 = Insert Into Array(array=w1516, index=w1527, new element=w1515) -> (w1523:i16[])
            n643 = Insert Into Array(array=w1517, index=w1526, new element=w1514) -> (w1522:i16[])
          }
          frame True {
            n644 = call <vilib>:"Amplitude and Phase Spectrum.vi"("dt"=w1528, "Signal (V)"=w1534) -> ("Amp Spectrum Mag (Vrms)"=→"?":dbl[])  [unwired: 1 in, 2 out]
            n645 = call <vilib>:"Amplitude and Phase Spectrum.vi"("dt"=w1528, "Signal (V)"=w1533) -> ("Amp Spectrum Mag (Vrms)"=→"?":dbl[])  [unwired: 1 in, 2 out]
            n646 = call <vilib>:"Amplitude and Phase Spectrum.vi"("dt"=w1528, "Signal (V)"=w1535) -> ("Amp Spectrum Mag (Vrms)"=→"?":dbl[])  [unwired: 1 in, 2 out]
            n647 = call <vilib>:"Amplitude and Phase Spectrum.vi"("dt"=w1528, "Signal (V)"=w1536) -> ("Amp Spectrum Mag (Vrms)"=→"?":dbl[])  [unwired: 1 in, 2 out]
          }
        }
        n648 = Add(x=w1510, y=w1492) -> (x+y=w1511:i32)
        "收包 3" <- w1511
        n649 = Tick Count (ms)() -> (millisecond timer value=w1502:u32)
        n650 = Subtract(x=w1502, y=w1503) -> (x-y=w1501:u32)
        n651 = Subtract(x=w1511, y=w1510) -> (x-y=w1509:i32)
        n652 = Add(x=w1509, y=w1508) -> (x+y=w1504:i32)
        n653 = Add(x=w1498, y=w1501) -> (x+y=w1499:u32)
        n654 = Greater Or Equal?(x=w1504, y=1000000) -> (x >= y?=w1506:bool)
        n655 = Or(x=w1478, y=w1477) -> (x .or. y?=w1476:bool)
        n656 = case shown="真" w1506 {
          tunnel: [w1886 0] -> w1505
          tunnel: w1504 -> [w1886 w1889]
          tunnel: [w1885 u32 0] -> w1500
          tunnel: w1499 -> [w1885 w1890]
          frame False {
          }
          frame True {
            n657 = Divide(x=w1889, y=w1890) -> (x/y=→"KB/s 3":dbl)
          }
        }
      }
    }
  }
  n658 = while {
    tunnel: w2 -> [w1944]
    tunnel: w3 -> [w1943]
    tunnel: w1 -> [w1929]
    tunnel: w4 -> [w1942]
    stop <- FALSE stop-if-true
    n659 = Split 1D Array(array=w1929, index=1 ("索引")) -> (first subarray=w1927:u8[], second subarray=w1923:u8[])
    n660 = Split 1D Array(array=w1923, index=1 ("索引")) -> (first subarray=w1903:u8[], second subarray=w1922:u8[])
    n661 = Split 1D Array(array=w1922, index=1 ("索引")) -> (first subarray=w1902:u8[], second subarray=w1921:u8[])
    n662 = Split 1D Array(array=w1921, index=1 ("索引")) -> (first subarray=w1901:u8[], second subarray=w1900:u8[])
    n663 = flat-sequence {
      tunnel: [w1947] -> w1893
      tunnel: w1893 -> [w1952]
      tunnel: [w1950] -> w1892
      frame #0 {
        n664 = Wait (ms)(milliseconds to wait=u32 1000 ("毫秒倍数")) -> ()  [unwired: 1 out]
      }
      frame #1 {
        n665 = TCP Open Connection(address="192.168.1.18" ("名称"), remote port or service name=u16 3858 ("端口")) -> (connection ID=w1947:refnum<k5>)  [unwired: 3 in, 1 out]
      }
      frame #2 {
        n666 = TCP Write(connection ID=w1952, data in="INTxxxxx" ("数据输入")) -> (connection ID out=w1951:refnum<k5>)  [unwired: 2 in, 2 out]
        n667 = while {
          tunnel: w1951 -> [w1961]
          tunnel: [w1955] -> w1950
          stop <- w1956 stop-if-true
          n668 = TCP Read(connection ID=w1961, bytes to read=8 ("读取的字节")) -> (connection ID out=w1955:refnum<k5>, data out=w1959:string)  [unwired: 3 in, 1 out]
          n669 = String Subset(string=w1959, length (rest)=3 ("偏移量(0)")) -> (substring=w1958:string)  [unwired: 1 in]
          n670 = Equal?(x=w1958, y="ACK") -> (x = y?=w1956:bool)
        }
      }
    }
    n671 = Byte Array To String(unsigned byte array=w1927) -> (string=w1932:string)
    n672 = Byte Array To String(unsigned byte array=u8[] [3] ("无符号字节数组")) -> (string=w1909:string)
    n673 = Byte Array To String(unsigned byte array=u8[] [1] ("无符号字节数组")) -> (string=w1917:string)
    n674 = Byte Array To String(unsigned byte array=w1901) -> (string=w1911:string)
    n675 = Byte Array To String(unsigned byte array=w1903) -> (string=w1920:string)
    n676 = Concatenate Strings("PRExxxx" ("数据输入"), w1932) -> (w1930:string)
    n677 = Concatenate Strings("DIVxxx" ("数据输入"), w1917, w1920) -> (w1919:string)
    n678 = Concatenate Strings("DIVxxx" ("数据输入"), w1909, w1911) -> (w1894:string)
    n679 = TCP Write(connection ID=w1892, data in=w1930) -> (connection ID out=w1941:refnum<k5>)  [unwired: 2 in, 2 out]
    n680 = while {
      tunnel: w1941 -> [w2001]
      tunnel: [w1995] -> w1936
      stop <- w1996 stop-if-true
      n681 = TCP Read(connection ID=w2001, bytes to read=8 ("读取的字节")) -> (connection ID out=w1995:refnum<k5>, data out=w1999:string)  [unwired: 3 in, 1 out]
      n682 = String Subset(string=w1999, length (rest)=3 ("偏移量(0)")) -> (substring=w1998:string)  [unwired: 1 in]
      n683 = Equal?(x=w1998, y="ACK") -> (x = y?=w1996:bool)
    }
    n684 = TCP Write(connection ID=w1936, data in=w1919) -> (connection ID out=w1940:refnum<k5>)  [unwired: 2 in, 2 out]
    n685 = while {
      tunnel: w1940 -> [w1993]
      tunnel: [w1987] -> w1935
      stop <- w1988 stop-if-true
      n686 = TCP Read(connection ID=w1993, bytes to read=8 ("读取的字节")) -> (connection ID out=w1987:refnum<k5>, data out=w1991:string)  [unwired: 3 in, 1 out]
      n687 = String Subset(string=w1991, length (rest)=3 ("偏移量(0)")) -> (substring=w1990:string)  [unwired: 1 in]
      n688 = Equal?(x=w1990, y="ACK") -> (x = y?=w1988:bool)
    }
    n689 = Byte Array To String(unsigned byte array=u8[] [4] ("无符号字节数组")) -> (string=w1905:string)
    n690 = Byte Array To String(unsigned byte array=w1900) -> (string=w1907:string)
    n691 = Byte Array To String(unsigned byte array=u8[] [2] ("无符号字节数组")) -> (string=w1913:string)
    n692 = Byte Array To String(unsigned byte array=w1902) -> (string=w1915:string)
    n693 = Concatenate Strings("DIVxxx" ("数据输入"), w1905, w1907) -> (w1898:string)
    n694 = Concatenate Strings("DIVxxx" ("数据输入"), w1913, w1915) -> (w1899:string)
    n695 = TCP Write(connection ID=w1935, data in=w1899) -> (connection ID out=w1939:refnum<k5>)  [unwired: 2 in, 2 out]
    n696 = while {
      tunnel: w1939 -> [w1985]
      tunnel: [w1979] -> w1934
      stop <- w1980 stop-if-true
      n697 = TCP Read(connection ID=w1985, bytes to read=8 ("读取的字节")) -> (connection ID out=w1979:refnum<k5>, data out=w1983:string)  [unwired: 3 in, 1 out]
      n698 = String Subset(string=w1983, length (rest)=3 ("偏移量(0)")) -> (substring=w1982:string)  [unwired: 1 in]
      n699 = Equal?(x=w1982, y="ACK") -> (x = y?=w1980:bool)
    }
    n700 = TCP Write(connection ID=w1934, data in=w1894) -> (connection ID out=w1938:refnum<k5>)  [unwired: 2 in, 2 out]
    n701 = while {
      tunnel: w1938 -> [w1977]
      tunnel: [w1971] -> w1933
      stop <- w1972 stop-if-true
      n702 = TCP Read(connection ID=w1977, bytes to read=8 ("读取的字节")) -> (connection ID out=w1971:refnum<k5>, data out=w1975:string)  [unwired: 3 in, 1 out]
      n703 = String Subset(string=w1975, length (rest)=3 ("偏移量(0)")) -> (substring=w1974:string)  [unwired: 1 in]
      n704 = Equal?(x=w1974, y="ACK") -> (x = y?=w1972:bool)
    }
    n705 = TCP Write(connection ID=w1933, data in=w1898) -> (connection ID out=w1937:refnum<k5>)  [unwired: 2 in, 2 out]
    n706 = while {
      tunnel: w1937 -> [w1969]
      tunnel: [w1963] -> w1897
      stop <- w1964 stop-if-true
      n707 = TCP Read(connection ID=w1969, bytes to read=8 ("读取的字节")) -> (connection ID out=w1963:refnum<k5>, data out=w1967:string)  [unwired: 3 in, 1 out]
      n708 = String Subset(string=w1967, length (rest)=3 ("偏移量(0)")) -> (substring=w1966:string)  [unwired: 1 in]
      n709 = Equal?(x=w1966, y="ACK") -> (x = y?=w1964:bool)
    }
    n710 = TCP Write(connection ID=w1897, data in="STAxxxxx" ("数据输入")) -> (connection ID out=w1895:refnum<k5>)  [unwired: 2 in, 2 out]
    n711 = while {
      tunnel: w1895 -> [w2050]
      tunnel: w1944 -> [w2049]
      tunnel: w1943 -> [w2022]
      tunnel: w1942 -> [w2002]
      stop <- w2012 stop-if-true
      n712 = Get Date/Time String(want seconds? (F)=TRUE ("需要秒？(F)")) -> (date string=w2020:string, time string=w2017:string)  [unwired: 2 in]
      n713 = Concatenate Strings(w2020, "-" ("字符串"), w2017, ".bin" ("字符串")) -> (w2016:string)
      n714 = Path To String(path=w2022) -> (string=w2033:string)
      n715 = Search and Replace String(replace all?=TRUE ("替换全部？(F)"), input string=w2016, search string=":" ("搜索字符串"), replace string="-" ("替换字符串(\"\")")) -> (result string=w2008:string)  [unwired: 4 in, 3 out]
      n716 = Search and Replace String(replace all?=TRUE ("替换全部？(F)"), input string=w2008, search string="/" ("搜索字符串"), replace string="-" ("替换字符串(\"\")")) -> (result string=w2007:string)  [unwired: 4 in, 3 out]
      n717 = Concatenate Strings(w2033, "\\2振动2-" ("字符串"), w2007) -> (w2040:string)
      n718 = Concatenate Strings(w2033, "\\2振动1-" ("字符串"), w2007) -> (w2039:string)
      n719 = Concatenate Strings(w2033, "\\2振动4-" ("字符串"), w2007) -> (w2042:string)
      n720 = Concatenate Strings(w2033, "\\2振动3-" ("字符串"), w2007) -> (w2041:string)
      n721 = Concatenate Strings(w2033, "\\2转速-" ("字符串"), w2007) -> (w2043:string)
      n722 = String To Path(string=w2040) -> (path=w2037:path)
      n723 = String To Path(string=w2041) -> (path=w2036:path)
      n724 = String To Path(string=w2039) -> (path=w2038:path)
      n725 = String To Path(string=w2042) -> (path=w2035:path)
      n726 = String To Path(string=w2043) -> (path=w2034:path)
      n727 = Open/Create/Replace File(file path (use dialog)=w2035, operation (0:open)=T1."open or create" ("操作(0:open)")) -> (refnum out=w2024:refnum<file>)  [unwired: 4 in, 2 out]
      n728 = Open/Create/Replace File(file path (use dialog)=w2037, operation (0:open)=T1."open or create" ("操作(0:open)")) -> (refnum out=w2026:refnum<file>)  [unwired: 4 in, 2 out]
      n729 = Open/Create/Replace File(file path (use dialog)=w2036, operation (0:open)=T1."open or create" ("操作(0:open)")) -> (refnum out=w2025:refnum<file>)  [unwired: 4 in, 2 out]
      n730 = Open/Create/Replace File(file path (use dialog)=w2034, operation (0:open)=T1."open or create" ("操作(0:open)")) -> (refnum out=w2023:refnum<file>)  [unwired: 4 in, 2 out]
      n731 = Open/Create/Replace File(file path (use dialog)=w2038, operation (0:open)=T1."open or create" ("操作(0:open)")) -> (refnum out=w2027:refnum<file>)  [unwired: 4 in, 2 out]
      n732 = while {
        shift-right: [w2108] -> _
        shift-left: _ -> [w2107]
        shift-right: [w2090] -> _
        shift-left: w2050 -> [w2094]
        shift-right: [w2102] -> _
        shift-left: _ -> [w2105]
        shift-right: [w2099] -> _
        shift-left: _ -> [w2100]
        shift-right: [w2097] -> _
        shift-left: _ -> [w2095]
        shift-right: [w2086] -> _
        shift-left: w2027 -> [w2081]
        shift-right: [w2085] -> _
        shift-left: w2026 -> [w2080]
        shift-right: [w2084] -> _
        shift-left: w2025 -> [w2079]
        shift-right: [w2083] -> _
        shift-left: w2024 -> [w2078]
        shift-right: [w2082] -> _
        shift-left: w2023 -> [w2077]
        tunnel: w2049 -> [w2076]
        tunnel: [w2074] -> w2012
        shift-right: [w2058] -> _
        shift-left: i16[] [] -> [w2062]
        shift-right: [w2059] -> _
        shift-left: i16[] [] -> [w2063]
        shift-right: [w2060] -> _
        shift-left: i16[] [] -> [w2064]
        shift-right: [w2061] -> _
        shift-left: i16[] [] -> [w2057]
        tunnel: w2002 -> [w2053]
        i -> [w2072]
        stop <- w2073 stop-if-true
        n733 = TCP Read(connection ID=w2094, bytes to read=1 ("读取的字节")) -> (connection ID out=w2087:refnum<k5>, data out=w2092:string)  [unwired: 3 in, 1 out]
        n734 = Equal?(x=w2092, y="D") -> (x = y?=w2088:bool)
        n735 = case shown="真" w2088 {
          tunnel: w2087 -> [w2150 w2171]
          tunnel: [w2150 w2170] -> w2090
          tunnel: [0 w2169] -> w2089
          tunnel: [FALSE w2167] -> w2074
          tunnel: [w2147 w2166] -> w2086
          tunnel: [w2146 w2159] -> w2085
          tunnel: [w2145 w2158] -> w2084
          tunnel: [w2144 w2157] -> w2083
          tunnel: [w2143 w2165] -> w2082
          tunnel: w2081 -> [w2147 w2164]
          tunnel: w2080 -> [w2146 w2163]
          tunnel: w2079 -> [w2145 w2162]
          tunnel: w2078 -> [w2144 w2161]
          tunnel: w2077 -> [w2143 w2160]
          tunnel: w2076 -> [_ w2156]
          tunnel: [FALSE w2155] -> w2075
          tunnel: [i16[] [] w2154] -> w2068
          tunnel: [i16[] [] w2153] -> w2067
          tunnel: [i16[] [] w2152] -> w2066
          tunnel: [i16[] [] w2151] -> w2065
          frame False {
          }
          frame True {
            n736 = TCP Read(connection ID=w2171, bytes to read=1 ("读取的字节")) -> (connection ID out=w2168:refnum<k5>, data out=w2174:string)  [unwired: 3 in, 1 out]
            n737 = Equal?(x=w2174, y="A") -> (x = y?=w2172:bool)
            n738 = case shown="真" w2172 {
              tunnel: w2168 -> [w2188 w2209]
              tunnel: [w2188 w2208] -> w2170
              tunnel: [0 w2207] -> w2169
              tunnel: [FALSE w2205] -> w2167
              tunnel: [w2185 w2204] -> w2166
              tunnel: [w2181 w2200] -> w2165
              tunnel: w2164 -> [w2185 w2199]
              tunnel: w2163 -> [w2184 w2198]
              tunnel: w2162 -> [w2183 w2197]
              tunnel: w2161 -> [w2182 w2196]
              tunnel: w2160 -> [w2181 w2195]
              tunnel: [w2184 w2203] -> w2159
              tunnel: [w2183 w2202] -> w2158
              tunnel: [w2182 w2201] -> w2157
              tunnel: w2156 -> [_ w2194]
              tunnel: [FALSE w2193] -> w2155
              tunnel: [i16[] [] w2192] -> w2154
              tunnel: [i16[] [] w2191] -> w2153
              tunnel: [i16[] [] w2190] -> w2152
              tunnel: [i16[] [] w2189] -> w2151
              frame False {
              }
              frame True {
                n739 = TCP Read(connection ID=w2209, bytes to read=1 ("读取的字节")) -> (connection ID out=w2206:refnum<k5>, data out=w2212:string)  [unwired: 3 in, 1 out]
                n740 = Equal?(x=w2212, y="T") -> (x = y?=w2210:bool)
                n741 = case shown="真" w2210 {
                  tunnel: w2206 -> [w2226 w2248]
                  tunnel: [w2226 w2245] -> w2208
                  tunnel: [0 w2247] -> w2207
                  tunnel: [FALSE w2244] -> w2205
                  tunnel: [w2219 w2236] -> w2204
                  tunnel: [w2220 w2235] -> w2203
                  tunnel: [w2221 w2234] -> w2202
                  tunnel: [w2222 w2243] -> w2201
                  tunnel: [w2223 w2242] -> w2200
                  tunnel: w2199 -> [w2219 w2241]
                  tunnel: w2198 -> [w2220 w2240]
                  tunnel: w2197 -> [w2221 w2239]
                  tunnel: w2196 -> [w2222 w2238]
                  tunnel: w2195 -> [w2223 w2237]
                  tunnel: w2194 -> [_ w2233]
                  tunnel: [FALSE w2232] -> w2193
                  tunnel: [i16[] [] w2231] -> w2192
                  tunnel: [i16[] [] w2230] -> w2191
                  tunnel: [i16[] [] w2229] -> w2190
                  tunnel: [i16[] [] w2228] -> w2189
                  frame False {
                  }
                  frame True {
                    n742 = TCP Read(connection ID=w2248, bytes to read=2 ("读取的字节")) -> (connection ID out=w2246:refnum<k5>)  [unwired: 3 in, 2 out]
                    n743 = case shown="真" TRUE {
                      tunnel: w2246 -> [w2262 w2398]
                      tunnel: [0 w2389] -> w2247
                      tunnel: [w2262 w2382] -> w2245
                      tunnel: [FALSE w2383] -> w2244
                      tunnel: [w2256 w2365] -> w2243
                      tunnel: [w2255 w2364] -> w2242
                      tunnel: w2241 -> [w2259 w2371]
                      tunnel: w2240 -> [w2258 w2369]
                      tunnel: w2239 -> [w2257 w2367]
                      tunnel: w2238 -> [w2256 w2291]
                      tunnel: w2237 -> [w2255 w2363]
                      tunnel: [w2259 w2370] -> w2236
                      tunnel: [w2258 w2368] -> w2235
                      tunnel: [w2257 w2366] -> w2234
                      tunnel: w2233 -> [_ w2361]
                      tunnel: [FALSE w2359] -> w2232
                      tunnel: [i16[] [] w2290] -> w2231
                      tunnel: [i16[] [] w2289] -> w2230
                      tunnel: [i16[] [] w2288] -> w2229
                      tunnel: [i16[] [] w2287] -> w2228
                      frame False {
                      }
                      frame True {
                        n744 = TCP Read(connection ID=w2398, bytes to read=4021 ("最大值(548)")) -> (connection ID out=w2372:refnum<k5>, data out=w2381:string)  [unwired: 3 in, 1 out]
                        n745 = String To Byte Array(string=w2381) -> (unsigned byte array=w2380:u8[])
                        n746 = String Length(string=w2381) -> (length=w2389:i32)
                        n747 = Split 1D Array(array=w2380, index=1000 ("索引")) -> (first subarray=w2285:u8[], second subarray=w2282:u8[])
                        n748 = Split 1D Array(array=w2282, index=1000 ("索引")) -> (first subarray=w2281:u8[], second subarray=w2278:u8[])
                        n749 = Split 1D Array(array=w2278, index=1000 ("索引")) -> (first subarray=w2277:u8[], second subarray=w2276:u8[])
                        n750 = Split 1D Array(array=w2276, index=1000 ("索引")) -> (first subarray=w2273:u8[], second subarray=w2286:u8[])
                        n751 = Split 1D Array(array=w2286, index=2 ("索引")) -> (first subarray=w2268:u8[], second subarray=w2358:u8[])
                        n752 = Split 1D Array(array=w2358, index=2 ("索引")) -> (first subarray=w2341:u8[], second subarray=w2357:u8[])
                        n753 = Split 1D Array(array=w2357, index=2 ("索引")) -> (first subarray=w2305:u8[], second subarray=w2356:u8[])
                        n754 = Split 1D Array(array=w2356, index=2 ("索引")) -> (first subarray=w2304:u8[], second subarray=w2343:u8[])
                        n755 = Split 1D Array(array=w2343, index=2 ("索引")) -> (first subarray=w2303:u8[], second subarray=w2352:u8[])
                        n756 = Split 1D Array(array=w2352, index=2 ("索引")) -> (first subarray=w2302:u8[], second subarray=w2351:u8[])
                        n757 = Split 1D Array(array=w2351, index=2 ("索引")) -> (first subarray=w2301:u8[], second subarray=w2342:u8[])
                        n758 = Split 1D Array(array=w2342, index=2 ("索引")) -> (first subarray=w2300:u8[], second subarray=w2264:u8[])
                        n759 = Split 1D Array(array=w2264, index=5 ("索引")) -> (first subarray=w2263:u8[])  [unwired: 1 out]
                        n760 = Decimate 1D Array(w2285) -> (w2284:u8[], w2283:u8[])
                        n761 = Decimate 1D Array(w2281) -> (w2280:u8[], w2279:u8[])
                        n762 = Decimate 1D Array(w2268) -> (w2270:u8[], w2269:u8[])
                        n763 = Decimate 1D Array(w2277) -> (w2275:u8[], w2274:u8[])
                        n764 = Decimate 1D Array(w2273) -> (w2272:u8[], w2271:u8[])
                        n765 = Get Date/Time String(date format (0)=enum16{"short", "long", "abbreviated"}."short" ("日期格式(0)"), want seconds? (F)=TRUE ("需要秒？(F)")) -> (date string=w2377:string, time string=w2360:string)  [unwired: 1 in]
                        n766 = Join Numbers(hi=w2270, lo=w2269) -> ((hi.lo)=w2267:u16[])
                        n767 = Join Numbers(hi=w2284, lo=w2283) -> ((hi.lo)=w2396:u16[])
                        n768 = Join Numbers(hi=w2280, lo=w2279) -> ((hi.lo)=w2391:u16[])
                        n769 = Join Numbers(hi=w2275, lo=w2274) -> ((hi.lo)=w2392:u16[])
                        n770 = Join Numbers(hi=w2272, lo=w2271) -> ((hi.lo)=w2393:u16[])
                        n771 = Index Array(array=w2341, index=0 ("索引")) -> (element=w2336:u8)
                        n772 = Index Array(array=w2341, index=1 ("索引")) -> (element=w2338:u8)
                        n773 = String To Byte Array(string="_PSAI") -> (unsigned byte array=w2386:u8[])
                        n774 = Index Array(array=w2305, index=0 ("索引")) -> (element=w2330:u8)
                        n775 = Index Array(array=w2305, index=1 ("索引")) -> (element=w2332:u8)
                        n776 = Index Array(array=w2303, index=0 ("索引")) -> (element=w2318:u8)
                        n777 = Index Array(array=w2304, index=0 ("索引")) -> (element=w2324:u8)
                        n778 = Index Array(array=w2303, index=1 ("索引")) -> (element=w2320:u8)
                        n779 = Index Array(array=w2304, index=1 ("索引")) -> (element=w2326:u8)
                        n780 = Index Array(array=w2302, index=0 ("索引")) -> (element=w2312:u8)
                        n781 = To Word Integer(number=w2396) -> (16bit integer=w2290:i16[])
                        "?" <- w2290
                        n782 = To Word Integer(number=w2267) -> (16bit integer=w2266:i16[])
                        "?" <- w2266
                        n783 = Index Array(array=w2302, index=1 ("索引")) -> (element=w2314:u8)
                        n784 = To Word Integer(number=w2391) -> (16bit integer=w2289:i16[])
                        "?" <- w2289
                        n785 = Index Array(array=w2301, index=0 ("索引")) -> (element=w2306:u8)
                        n786 = call <vilib>:"Space Constant.vi"() -> ("String"=w2373:string)
                        n787 = Index Array(array=w2301, index=1 ("索引")) -> (element=w2308:u8)
                        n788 = To Word Integer(number=w2392) -> (16bit integer=w2288:i16[])
                        "?" <- w2288
                        n789 = To Word Integer(number=w2393) -> (16bit integer=w2287:i16[])
                        "?" <- w2287
                        n790 = Equal?(x=w2263, y=w2386) -> (x = y?=w2385:bool[])
                        n791 = Index Array(array=w2300, index=0 ("索引")) -> (element=→"?":u8)
                        n792 = Divide(x=w2338, y=10.0) -> (x/y=w2337:dbl)
                        n793 = Divide(x=w2332, y=10.0) -> (x/y=w2331:dbl)
                        n794 = Divide(x=w2320, y=10.0) -> (x/y=w2319:dbl)
                        n795 = Divide(x=w2326, y=10.0) -> (x/y=w2325:dbl)
                        n796 = Concatenate Strings("\r", "@@" ("字符串"), w2377, w2373, w2360, "@@" ("字符串")) -> (w2376:string)
                        "系统时间 4" <- w2376
                        n797 = Divide(x=w2314, y=10.0) -> (x/y=w2313:dbl)
                        n798 = Index Array(array=w2300, index=1 ("索引")) -> (element=→"?":u8)
                        n799 = Divide(x=w2308, y=10.0) -> (x/y=w2307:dbl)
                        n800 = And Array Elements(Boolean array=w2385) -> (logical AND=w2384:bool)
                        n801 = Add(x=w2336, y=w2337) -> (x+y=→"?":dbl)
                        n802 = Add(x=w2330, y=w2331) -> (x+y=→"?":dbl)
                        n803 = Add(x=w2318, y=w2319) -> (x+y=→"?":dbl)
                        n804 = Add(x=w2324, y=w2325) -> (x+y=→"?":dbl)
                        n805 = Add(x=w2312, y=w2313) -> (x+y=→"?":dbl)
                        n806 = Add(x=w2306, y=w2307) -> (x+y=→"?":dbl)
                        n807 = local write "系统时间 4"(w2376) -> ()
                        n808 = case shown="真" w2384 {
                          tunnel: [w2408 w2427] -> w2382
                          tunnel: [TRUE FALSE] -> w2383
                          tunnel: w2372 -> [w2406 w2427]
                          tunnel: w2290 -> [_ w2426]
                          tunnel: w2289 -> [_ w2425]
                          tunnel: w2288 -> [_ w2424]
                          tunnel: w2287 -> [_ w2423]
                          tunnel: w2266 -> [_ w2422]
                          tunnel: w2371 -> [w2404 w2420]
                          tunnel: [w2404 w2419] -> w2370
                          tunnel: w2369 -> [w2405 w2418]
                          tunnel: [w2405 w2417] -> w2368
                          tunnel: w2367 -> [w2403 w2416]
                          tunnel: [w2403 w2415] -> w2366
                          tunnel: w2291 -> [w2402 w2414]
                          tunnel: [w2402 w2413] -> w2365
                          tunnel: [w2401 w2412] -> w2364
                          tunnel: w2363 -> [w2401 w2411]
                          tunnel: w2361 -> [_ w2410]
                          tunnel: [FALSE w2409] -> w2359
                          frame False {
                            n809 = TCP Close Connection(connection ID=w2406) -> (connection ID out=w2408:refnum<k5>)  [unwired: 2 in, 1 out]
                          }
                          frame True {
                            n810 = case shown="真" w2410 {
                              tunnel: w2426 -> [_ w2480]
                              tunnel: w2425 -> [_ w2460]
                              tunnel: w2424 -> [_ w2459]
                              tunnel: w2423 -> [_ w2458]
                              tunnel: w2422 -> [_ w2457]
                              tunnel: w2420 -> [w2433 w2446]
                              tunnel: [w2433 w2437] -> w2419
                              tunnel: w2418 -> [w2432 w2445]
                              tunnel: [w2432 w2444] -> w2417
                              tunnel: w2416 -> [w2431 w2443]
                              tunnel: [w2431 w2438] -> w2415
                              tunnel: w2414 -> [w2430 w2442]
                              tunnel: [w2430 w2441] -> w2413
                              tunnel: [w2429 w2440] -> w2412
                              tunnel: w2411 -> [w2429 w2439]
                              tunnel: [FALSE w2434] -> w2409
                              frame False {
                              }
                              frame True {
                                n811 = local read "系统时间 4"() -> (w2454:string)
                                n812 = local read "系统时间 4"() -> (w2456:string)
                                n813 = local read "系统时间 4"() -> (w2448:string)
                                n814 = local read "系统时间 4"() -> (w2450:string)
                                n815 = local read "系统时间 4"() -> (w2452:string)
                                n816 = String To Byte Array(string=w2454) -> (unsigned byte array=w2453:u8[])
                                n817 = String To Byte Array(string=w2450) -> (unsigned byte array=w2449:u8[])
                                n818 = String To Byte Array(string=w2448) -> (unsigned byte array=w2447:u8[])
                                n819 = String To Byte Array(string=w2456) -> (unsigned byte array=w2455:u8[])
                                n820 = String To Byte Array(string=w2452) -> (unsigned byte array=w2451:u8[])
                                n821 = Insert Into Array(array=w2480, index=0 ("索引"), new element=w2447) -> (w2478:i16[])
                                n822 = Insert Into Array(array=w2460, index=0 ("索引"), new element=w2449) -> (w2474:i16[])
                                n823 = Insert Into Array(array=w2459, index=0 ("索引"), new element=w2451) -> (w2470:i16[])
                                n824 = Insert Into Array(array=w2458, index=0 ("索引"), new element=w2453) -> (w2466:i16[])
                                n825 = Insert Into Array(array=w2457, index=0 ("索引"), new element=w2455) -> (w2462:i16[])
                                n826 = Write to Binary File(file (use dialog)=w2446, data=w2478, 5:FALSE ("预置数组或字符串大小？(T)"), 9:T2."little-endian" ("字节顺序(0:big-endian, network order)")) -> (refnum out=w2437:refnum<file>)  [unwired: 2 in, 2 out]
                                n827 = Write to Binary File(file (use dialog)=w2445, data=w2474, 5:FALSE ("预置数组或字符串大小？(T)"), 9:T2."little-endian" ("字节顺序(0:big-endian, network order)")) -> (refnum out=w2444:refnum<file>)  [unwired: 2 in, 2 out]
                                n828 = Write to Binary File(file (use dialog)=w2443, data=w2470, 5:FALSE ("预置数组或字符串大小？(T)"), 9:T2."little-endian" ("字节顺序(0:big-endian, network order)")) -> (refnum out=w2438:refnum<file>)  [unwired: 2 in, 2 out]
                                n829 = Write to Binary File(file (use dialog)=w2442, data=w2466, 5:FALSE ("预置数组或字符串大小？(T)"), 9:T2."little-endian" ("字节顺序(0:big-endian, network order)")) -> (refnum out=w2441:refnum<file>)  [unwired: 2 in, 2 out]
                                n830 = Write to Binary File(file (use dialog)=w2439, data=w2462, 5:FALSE ("预置数组或字符串大小？(T)"), 9:T2."little-endian" ("字节顺序(0:big-endian, network order)")) -> (refnum out=w2440:refnum<file>)  [unwired: 2 in, 2 out]
                                n831 = Get File Size(file=w2437) -> (size (in bytes)=w2436:i64)  [unwired: 1 in, 2 out]
                                n832 = Greater Or Equal?(x=w2436, y=i64 60000000) -> (x >= y?=w2434:bool)
                              }
                            }
                          }
                        }
                      }
                    }
                  }
                }
              }
            }
          }
        }
        n833 = Divide(x=u8 187, y=w2053) -> (x/y=w2051:dbl)
        n834 = Round Toward -Infinity(1:w2051) -> (0:w2055:dbl)
        n835 = Multiply(x=w2055, y=500.0) -> (x*y=w2054:dbl)
        n836 = Quotient & Remainder(x=w2072, y=w2055) -> (x-y*floor(x/y)=w2071:dbl)  [unwired: 1 out]
        n837 = Equal?(x=w2071, y=0) -> (x = y?=w2069:bool)
        n838 = case shown="真" w2069 {
          tunnel: w2068 -> [w2112 w2137]
          tunnel: w2067 -> [w2111 w2136]
          tunnel: w2066 -> [w2110 w2135]
          tunnel: w2065 -> [w2109 w2134]
          tunnel: [w2120 w2137] -> w2058
          tunnel: [w2119 w2136] -> w2059
          tunnel: [w2118 w2135] -> w2060
          tunnel: [w2117 w2134] -> w2061
          tunnel: w2057 -> [w2116 w2130]
          tunnel: w2064 -> [w2115 w2133]
          tunnel: w2063 -> [w2114 w2131]
          tunnel: w2062 -> [w2113 w2132]
          tunnel: w2054 -> [_ w2125]
          frame False {
            n839 = Array Size(array=w2115) -> (size(s)=w2122:i32)
            n840 = Array Size(array=w2116) -> (size(s)=w2121:i32)
            n841 = Array Size(array=w2113) -> (size(s)=w2124:i32)
            n842 = Array Size(array=w2114) -> (size(s)=w2123:i32)
            n843 = Insert Into Array(array=w2115, index=w2122, new element=w2110) -> (w2118:i16[])
            n844 = Insert Into Array(array=w2116, index=w2121, new element=w2109) -> (w2117:i16[])
            n845 = Insert Into Array(array=w2113, index=w2124, new element=w2112) -> (w2120:i16[])
            n846 = Insert Into Array(array=w2114, index=w2123, new element=w2111) -> (w2119:i16[])
          }
          frame True {
            n847 = call <vilib>:"Amplitude and Phase Spectrum.vi"("dt"=w2125, "Signal (V)"=w2131) -> ("Amp Spectrum Mag (Vrms)"=→"?":dbl[])  [unwired: 1 in, 2 out]
            n848 = call <vilib>:"Amplitude and Phase Spectrum.vi"("dt"=w2125, "Signal (V)"=w2130) -> ("Amp Spectrum Mag (Vrms)"=→"?":dbl[])  [unwired: 1 in, 2 out]
            n849 = call <vilib>:"Amplitude and Phase Spectrum.vi"("dt"=w2125, "Signal (V)"=w2132) -> ("Amp Spectrum Mag (Vrms)"=→"?":dbl[])  [unwired: 1 in, 2 out]
            n850 = call <vilib>:"Amplitude and Phase Spectrum.vi"("dt"=w2125, "Signal (V)"=w2133) -> ("Amp Spectrum Mag (Vrms)"=→"?":dbl[])  [unwired: 1 in, 2 out]
          }
        }
        n851 = Add(x=w2107, y=w2089) -> (x+y=w2108:i32)
        "收包 4" <- w2108
        n852 = Tick Count (ms)() -> (millisecond timer value=w2099:u32)
        n853 = Subtract(x=w2099, y=w2100) -> (x-y=w2098:u32)
        n854 = Subtract(x=w2108, y=w2107) -> (x-y=w2106:i32)
        n855 = Add(x=w2106, y=w2105) -> (x+y=w2101:i32)
        n856 = Add(x=w2095, y=w2098) -> (x+y=w2096:u32)
        n857 = Greater Or Equal?(x=w2101, y=1000000) -> (x >= y?=w2103:bool)
        n858 = Or(x=w2075, y=w2074) -> (x .or. y?=w2073:bool)
        n859 = case shown="真" w2103 {
          tunnel: [w2483 0] -> w2102
          tunnel: w2101 -> [w2483 w2486]
          tunnel: [w2482 u32 0] -> w2097
          tunnel: w2096 -> [w2482 w2487]
          frame False {
          }
          frame True {
            n860 = Divide(x=w2486, y=w2487) -> (x/y=→"KB/s 4":dbl)
          }
        }
      }
    }
  }
